vi "plcHMI_rev2.vi"() -> ()   [LabVIEW 2020]
doc: "ADS continuos synchronous write example using base blocks. \n\nThe client writes data synchronously and does wait for the respose from server."
uses:
  Agilent/AgilentTotalCluster.ctl
  Agilent/AgilentControl.ctl
  Agilent/Channel Config.ctl
  <vilib>/Platform/TimedLoop/XDataNode/timing_clust.ctl
  <vilib>/Platform/TimedLoop/XDataNode/nitl_modes.ctl
  <vilib>/Platform/TimedLoop/XDataNode/wakeup.ctl
  <userlib>/Beckhoff-LabVIEW-Interface/_DependsOn/With TypeResolving/Write Sync Single TypeResolved.vi
  <userlib>/Beckhoff-LabVIEW-Interface/_DependsOn/With TypeResolving/Read Sync Single TypeResolved.vi
  <vilib>/Platform/TimedLoop/XDataNode/XDataNode.xnode
  <vilib>/Platform/TimedLoop/XDataNode/XDNodeRunTimeDep.lvlib
panel:
  in  "Tab Control":T1(tab)
  out "error out":errorcluster
  in  "Symbol file path - MUST BE ENTERED\nLoad \"ADS Write AND Read Symbols REV X.X.xml\"":path
  out "bHasMached":bool
  out "Write Status":bool
  out "Read Status":bool
  in  "EXIT HMI":bool caption="STOP HMI\nEXIT HMI"
  out "Internal TwinCAT Handle ID Maps":dbl format="%#_12g"
  in  "802L TDK PSU Voltage Rating (abs(Volts))":i32=12000 min=1 max=50000
  in  "802L TDL PSU Peak Power (J/s)":i32=9000 min=1 max=50000
  in  "HVPS Model":u16(ring) items=["802L-12kV,9000J/s", "802L+50kV,9000J/s", "Other"]
  out "Test Interval Fault":bool
  in  "Cycle Time (Sec)":i32=15 min=0
  in  "Voltage Held by PSU":bool
  in  "Log Capacitor Voltage":bool
  in  "Log Temperature Data":bool
  out "Time Since Last Shot":string caption="Elapsed Time Text"
  in  "Duty Cycle":dbl
  in  "Current Control":bool
  out "Expected Voltage":i16
  in  "Dump":bool
  out "EOC":bool
  out "Maximum Test Number Reached":bool
  out "SCR Ready":bool
  in  "START":bool
  in  "STOP":bool
  in  "Hold":bool
  in  "Charge":bool
  in  "Shot":bool
  in  "HV Switch Mode":bool
  in  "CLEAR FAULT":bool
  in  "Manual/Auto":bool=TRUE
  out "Test Interval (Sec)":i32=15 min=0
  in  "Capacitance (uF)":sgl=1e-13 min=0 max=10000 format="%#_6f"
  in  "Target Charge Volt (V) - Min 1500V - TEMPORARY LIMIT 12kV":i32 min=-12000 max=12000 step=1
  out "Estimated Charge Time (seconds)":sgl
  in  "Hold Time Before Shot (seconds)":i16 min=0 max=1000
  in  "Max Number of Shots (Test intervals)":i32=1 min=1 max=999
  out "Shot Number":i32
  out "Charge Fault":bool=TRUE
  out "Discharge Fault":bool=TRUE
  out "Hold Fault":bool=TRUE
  out "Cap 1 Temp\nExceeded Fault":bool=TRUE
  out "Ambient Temp\nExceeded Fault":bool=TRUE
  out "PSU Fault":bool=TRUE
  out "Control Sys Fault":bool=TRUE
  out "test Running":bool
  out "Test State":string
  out "Cap 1 Voltage":i16
  out "Cap 1 Temperature":i16
  in  "Capacitor Voltage Data Log File Path (.xlsx)":path
  out "Load Temperature":i16
  out "Soft Dump Temp":i16
  out "Ambient Temp":i16
  out "Waveform Chart - Capacitor Voltage (Probe, abs(Volts))":dbl(graph)
  in  "Manual Charge Time (seconds)":sgl=-1.0 min=-1 max=90
  in  "Reset Test Number":bool
  in  "Cap 1 Fault Temp (Cel)":i16 min=0 max=125
  in  "Capacitor Temperature Data Log File Path (.xlsx)":path
  out "Cap 1 Voltage (HVPS)":i16
  out "Capacitor Voltage":cluster{dbl, dbl}(graph)
  out "EOC":i16(graph)
  out "Soft Exception":bool
  out "PSU HV FB Fault":bool
  out "Charge FB Fault":bool
  out "Softdump FB Fault":bool
  out "SCR FB":i16(graph)
  in  "CH4 Vertical Units":string(combo)="V"
  in  "CH4 Vertical Units/div":dbl=2.0
  in  "Toggle Scope Scale":bool
  in  "CH1 Vertical Units/div":dbl=2.0
  in  "CH1 Vertical Units":string(combo)="V"
  in  "Horizontal Units":enum16{"us", "ms", "s"}(ring)
  in  "Horizontal Units/div":dbl=200.0
  out "Download":bool
  in  "Single":bool
  in  "Stop":bool
  out "Scope Trig":bool
  in  "Agilent Array":T2[](array[typedef])
  out "Process Step":i32
  in  "C:\\HVTest\\Local_Cap_Log_Scope (.xlsx)":path
  out "Stop Loops":bool
  # "CONFIGURATION"
  # "Press STOP HMI instead of\nLabView Abort Execution"
  # "PSU V Rating, Peak Power\nactive when OTHER\nis selected"
  # "INPUT VARIABLES - For TDK Lambda 802L\nMust be written to before START"
  # "FAULT STATUSES"
  # "Set to -1 for automated\nfull charge to setpoint"
  # "MANUAL CONTROLS"
  # "Does not record during \"wait\" and appends to data file. Must be named with .xlsx"
  # "HV Switch Configuration"
  # "Records during \"Test Running.\" Must be named with .xlsx"
  # "Control Sys Faults"
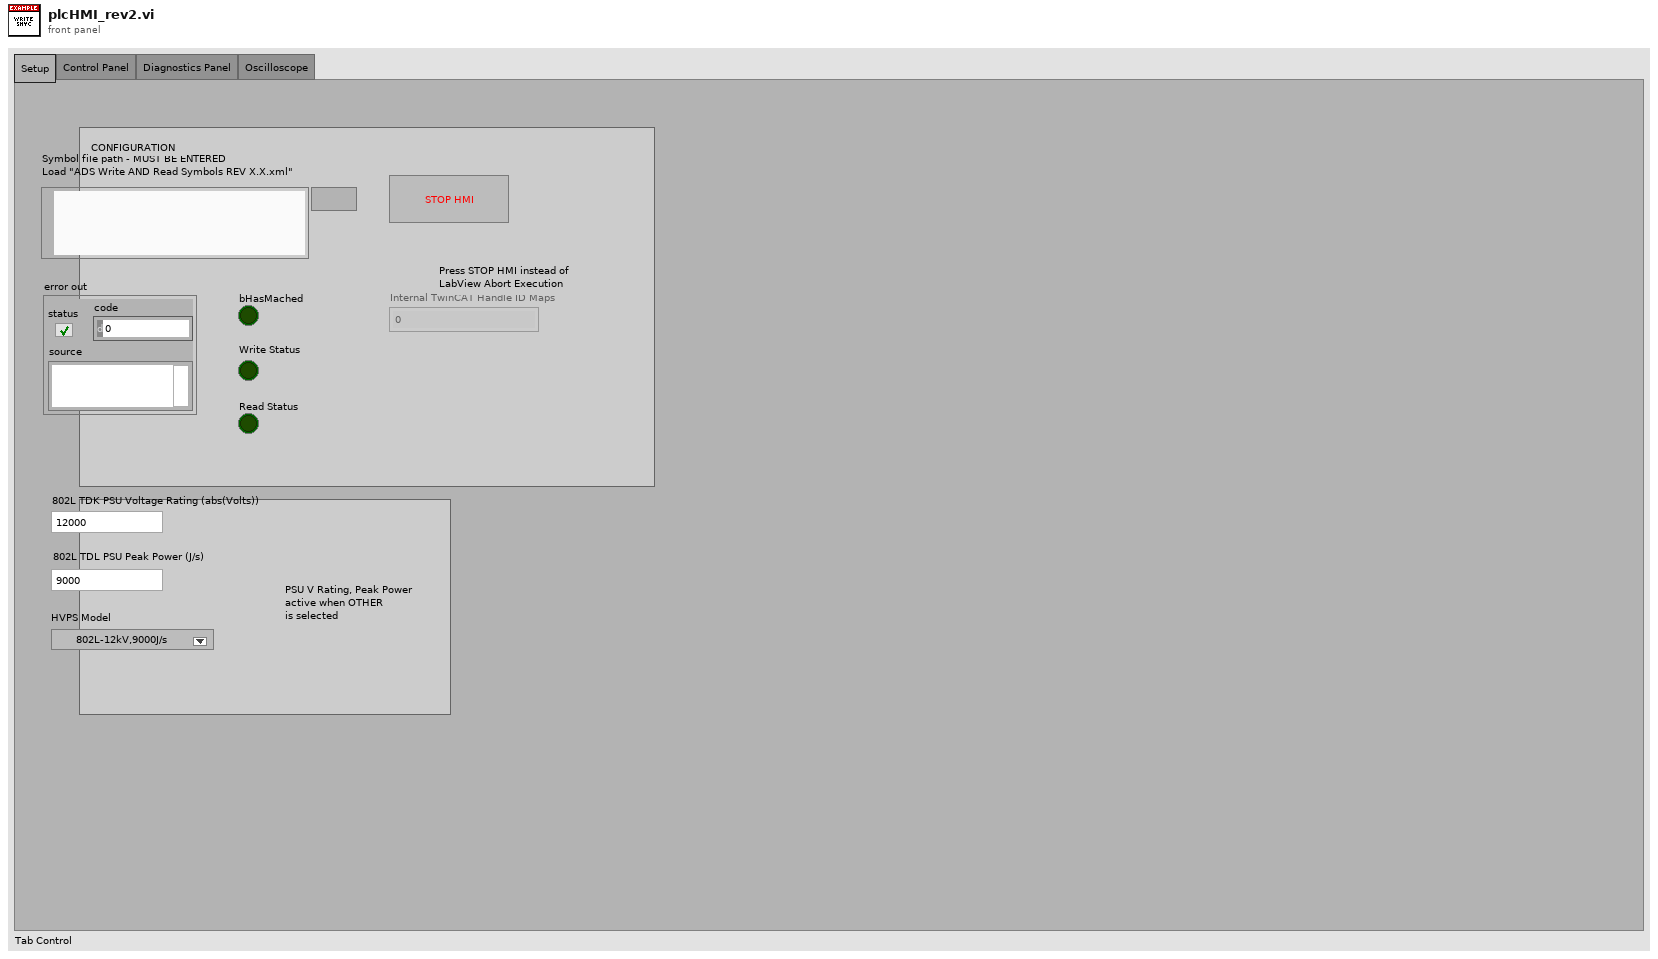
[diagram p1: front panel]
types:
  T1 = enum32{"Setup", "Control Panel", "Diagnostics Panel", "Oscilloscope"}
  T2 = typedef "AgilentTotalCluster.ctl" = cluster{"Agilent Graph":waveform(dbl)[], "Agilent Control":T3, "Agilent Setup Error":errorcluster, "Agilent Present":bool, "Enabled":bool}
  T3 = typedef "AgilentControl.ctl" = cluster{"Trig?":bool, "VISA session":refnum<visa-resource-name>, "Setup to Load":string, "Timeout (ms)":u32, "Desired Samp":enum32{"100", "250", "500", "1000", "2000", "5000", "10000", "20000", "50000", "100000", "200000", "500000", "1000000", "2000000", "4000000", "8000000"}, "Captured Samp":i32, "Desired Channels":T4[]}
  T4 = typedef "Channel Config.ctl" = cluster{"Chan Index":enum16{"Channel1", "Channel2", "Channel3", "Channel4", "MATH"}, "Name":string, "Samples":i32}
  T5 = typedef "XDNodeRunTimeDep.lvlib/timing_clust.ctl" = cluster{"Expected End [f-1]":u64, "Actual End [f-1]":u64, "Finished Late? [f-1]":bool, "Expected End [i-1]":u64, "Actual End [i-1]":u64, "Finished Late? [i-1]":bool, "Expected Start [i]":u64, "Actual Start [i]":u64, "Expected Start [f]":u64, "Actual Start [f]":u64, "Source Name":string, "Structure Name":string, "Period":i64, "Deadline":i64, "Offset":i64, "Start":i64, "Priority":i32, "Timeout":i32, "Mode":T6, "Wakeup Reason":T7, "Error":errorcluster, "Source Type":string, "Secondary Source Type":string, "Global End Time":u64, "Global Start Time":u64, "Frame Duration":u64, "Iteration Duration":u64, "Assigned CPU":i32, "I/O Scan Engine Mode":u32}
  T6 = typedef "XDNodeRunTimeDep.lvlib/nitl_modes.ctl" = enum32{"No Change", "Process missed periods, maintain original phase", "Discard missed periods, maintain original phase", "Process missed periods, ignore original phase", "Discard missed periods, ignore original phase"}
  T7 = typedef "XDNodeRunTimeDep.lvlib/wakeup.ctl" = enum32{"Normal", "Aborted", "Asynchronous wakeup", "Timing source error", "Timed loop error", "Timeout"}
  T8 = cluster{"Agilent Array[0]":T2, "Agilent Array[1]":T2, "Agilent Array[2]":T2, "Agilent Array[3]":T2, "Agilent Array[4]":T2, "Agilent Array[5]":T2, "Agilent Array[6]":T2, "Agilent Array[7]":T2, "Agilent Array[8]":T2}
  T9 = enum32{"100", "250", "500", "1000", "2000", "5000", "10000", "20000", "50000", "100000", "200000", "500000", "1000000", "2000000", "4000000", "8000000"}
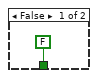
[diagram p2: hidden frame]
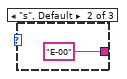
[diagram p5: hidden frame]
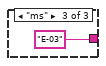
[diagram p6: hidden frame]
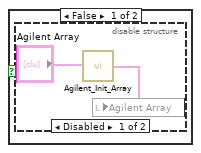
[diagram p7: hidden frame]
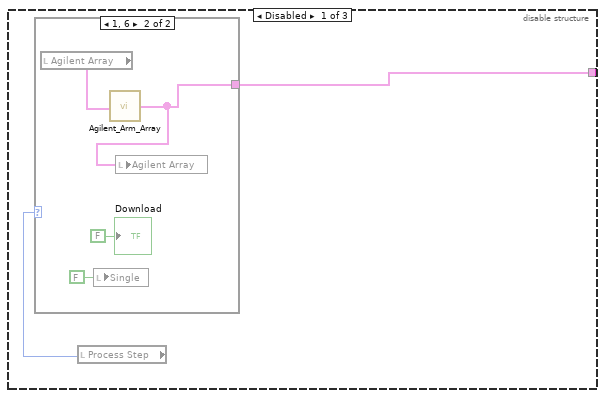
[diagram p11: hidden frame]
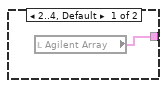
[diagram p12: hidden frame]
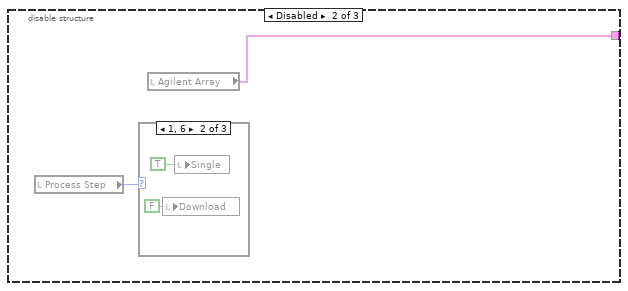
[diagram p13: hidden frame]
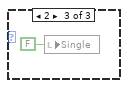
[diagram p15: hidden frame]
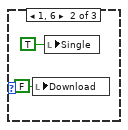
[diagram p17: hidden frame]
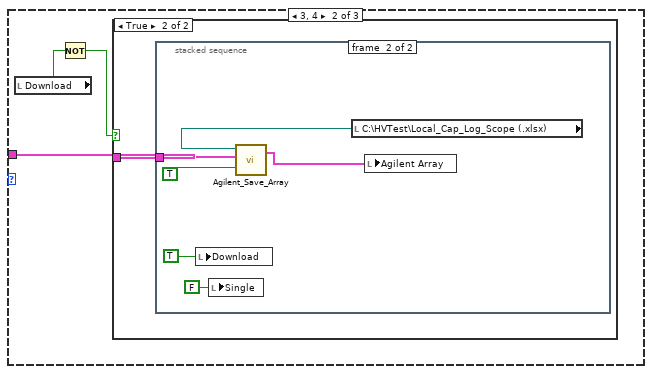
[diagram p19: hidden frame]
diagram:
  w95 = u16 17 items=["SyncLatest"=17, "AsyncLatest"=33] ("WriterMode")
  w188 = u16 33 items=["SyncLatest"=17, "AsyncLatest"=33] ("WriterMode")
  w227 = u16 33 items=["SyncLatest"=17, "AsyncLatest"=33] ("WriterMode")
  w246 = u16 33 items=["SyncLatest"=17, "AsyncLatest"=33] ("WriterMode")
  w265 = u16 33 items=["SyncLatest"=17, "AsyncLatest"=33] ("WriterMode")
  w284 = u16 33 items=["SyncLatest"=17, "AsyncLatest"=33] ("WriterMode")
  w303 = u16 33 items=["SyncLatest"=17, "AsyncLatest"=33] ("WriterMode")
  w322 = u16 33 items=["SyncLatest"=17, "AsyncLatest"=33] ("WriterMode")
  w341 = u16 17 items=["SyncLatest"=17, "AsyncLatest"=33] ("WriterMode")
  w360 = u16 17 items=["SyncLatest"=17, "AsyncLatest"=33] ("WriterMode")
  w379 = u16 17 items=["SyncLatest"=17, "AsyncLatest"=33] ("WriterMode")
  w398 = u16 17 items=["SyncLatest"=17, "AsyncLatest"=33] ("WriterMode")
  w417 = u16 17 items=["SyncLatest"=17, "AsyncLatest"=33] ("WriterMode")
  w436 = u16 17 items=["SyncLatest"=17, "AsyncLatest"=33] ("WriterMode")
  w455 = u16 17 items=["SyncLatest"=17, "AsyncLatest"=33] ("WriterMode")
  w470 = u16 17 items=["SyncLatest"=17, "AsyncLatest"=33] ("WriterMode")
  # "Variables/ Control"
  # "Documentation:\nCode separated vertically into two main sections - Write and read\nThey are further separated into BOOL and numeric\nThe OR gates wire all the error lines and the EXIT HMI button to a WHILE LOOP STOP\nThere current delay time on the routine is 100ms\nAll the AND gates connect the typecast resolve lines to the bHasMatched indicator\nThe second and third set of AND gates connect the write statuses to the Write Status indicator\nThe same is done for the read status indicator"
  # "WRITE NUMERICS"
  # "WRITE BOOLS"
  # "Select Symbol N"
  # "Read Initialization"
  # "Release \nTypeResolver"
  # "Release Writer"
  # "Send Request"
  # "Init \nTypeResolver"
  # "Init Writer"
  # "Select Symbol"
  # "Initialization"
  # "Call Release handle block\nat the end, when all nodes\nhave finished their execution"
  # "There must be only one release\nafter every init block.\nRelease block must be called\nalways at the end."
  # "Release"
  # "Symbol Interface"
  n1 = disable-structure shown="Enabled" {
    disable-tunnel: [w477 _] -> w475
    disable-tunnel: [w476 w479] -> w474
    frame Disabled {
      # "Using Symbol Interface"
      n2 = call <userlib>:"Symbol Interface.vi"() -> ("PortInfo"=w476:string, "error out"=w477:errorcluster)  [unwired: 14 in]
    }
    frame Enabled {
      # "Using Symbol File"
      n3 = Path To String(path="Symbol file path - MUST BE ENTERED\nLoad \"ADS Write AND Read Symbols REV X.X.xml\"") -> (string=w479:string)
    }
  }
  n4 = call <userlib>:"Init.vi"("XMLDescription"=w474, "error in (no error)"=w475) -> ("Handle"=w24:u32, "ReadGrpSymbols"=w5:string[], "WriteGrpSymbols"=w11:string[], "error out"=w16:errorcluster)  [unwired: 9 in, 1 out]
  n5 = Index Array(array=w11, index=21) -> (element=w10:string)
  n6 = Index Array(array=w11, index=20) -> (element=w17:string)
  n7 = Index Array(array=w11, index=14) -> (element=w228:string)
  n8 = Index Array(array=w11, index=9) -> (element=w323:string)
  n9 = Index Array(array=w11, index=10) -> (element=w304:string)
  n10 = Index Array(array=w11, index=12) -> (element=w266:string)
  n11 = Index Array(array=w11, index=11) -> (element=w285:string)
  n12 = Index Array(array=w11, index=13) -> (element=w247:string)
  n13 = Index Array(array=w11, index=18) -> (element=w25:string)
  n14 = Index Array(array=w11, index=19) -> (element=w18:string)
  n15 = Index Array(array=w11, index=7) -> (element=w342:string)
  n16 = Index Array(array=w11, index=2) -> (element=w437:string)
  n17 = Index Array(array=w11, index=3) -> (element=w418:string)
  n18 = Index Array(array=w11, index=5) -> (element=w380:string)
  n19 = Index Array(array=w11, index=4) -> (element=w399:string)
  n20 = Index Array(array=w11, index=6) -> (element=w361:string)
  n21 = Index Array(array=w11, index=1) -> (element=w456:string)
  n22 = Index Array(array=w11, index=16) -> (element=w122:string)
  n23 = Index Array(array=w11, index=8) -> (element=w94:string)
  n24 = Index Array(array=w11, index=0) -> (element=w471:string)
  n25 = Index Array(array=w11, index=15) -> (element=w189:string)
  n26 = Index Array(array=w11, index=17) -> (element=w78:string)
  n27 = call <userlib>:"Init Writer.vi"("Handle"=w24, "SymbolName"=w228, "WriterMode"=w227, "error constant"=w16) -> ("Handle"=w226:u32, "SymbolName"=w225:string, "WriterMode"=w224:u16, "WriteHandle"=w223:u32, "error IO"=w222:errorcluster)  [unwired: 7 in]
  n28 = call <userlib>:"Init Writer.vi"("Handle"=w24, "SymbolName"=w323, "WriterMode"=w322, "error constant"=w16) -> ("Handle"=w318:u32, "SymbolName"=w317:string, "WriterMode"=w316:u16, "WriteHandle"=w314:u32, "error IO"=w315:errorcluster)  [unwired: 7 in]
  n29 = call <userlib>:"Init Writer.vi"("Handle"=w24, "SymbolName"=w304, "WriterMode"=w303, "error constant"=w16) -> ("Handle"=w302:u32, "SymbolName"=w301:string, "WriterMode"=w300:u16, "WriteHandle"=w299:u32, "error IO"=w298:errorcluster)  [unwired: 7 in]
  n30 = call <userlib>:"Init Writer.vi"("Handle"=w24, "SymbolName"=w266, "WriterMode"=w265, "error constant"=w16) -> ("Handle"=w264:u32, "SymbolName"=w263:string, "WriterMode"=w262:u16, "WriteHandle"=w261:u32, "error IO"=w260:errorcluster)  [unwired: 7 in]
  n31 = call <userlib>:"Init Type.vi"("Handle"=w24, "SymbolName"=w228, "error in"=w16) -> ("Handle"=w221:u32, "TypeHdl"=w220:u32, "error IO"=w219:errorcluster)  [unwired: 7 in, 3 out]
  n32 = call <userlib>:"Init Type.vi"("Handle"=w24, "SymbolName"=w323, "error in"=w16) -> ("Handle"=w307:u32, "TypeHdl"=w306:u32, "error IO"=w305:errorcluster)  [unwired: 7 in, 3 out]
  n33 = call <userlib>:"Init Type.vi"("Handle"=w24, "SymbolName"=w304, "error in"=w16) -> ("Handle"=w297:u32, "TypeHdl"=w296:u32, "error IO"=w295:errorcluster)  [unwired: 7 in, 3 out]
  n34 = call <userlib>:"Init Writer.vi"("Handle"=w24, "SymbolName"=w285, "WriterMode"=w284, "error constant"=w16) -> ("Handle"=w283:u32, "SymbolName"=w282:string, "WriterMode"=w281:u16, "WriteHandle"=w280:u32, "error IO"=w279:errorcluster)  [unwired: 7 in]
  n35 = call <userlib>:"Init Type.vi"("Handle"=w24, "SymbolName"=w266, "error in"=w16) -> ("Handle"=w259:u32, "TypeHdl"=w258:u32, "error IO"=w257:errorcluster)  [unwired: 7 in, 3 out]
  n36 = call <userlib>:"Init Writer.vi"("Handle"=w24, "SymbolName"=w247, "WriterMode"=w246, "error constant"=w16) -> ("Handle"=w245:u32, "SymbolName"=w244:string, "WriterMode"=w243:u16, "WriteHandle"=w242:u32, "error IO"=w241:errorcluster)  [unwired: 7 in]
  n37 = call <userlib>:"Init Type.vi"("Handle"=w24, "SymbolName"=w285, "error in"=w16) -> ("Handle"=w278:u32, "TypeHdl"=w277:u32, "error IO"=w276:errorcluster)  [unwired: 7 in, 3 out]
  n38 = call <userlib>:"Init Type.vi"("Handle"=w24, "SymbolName"=w247, "error in"=w16) -> ("Handle"=w240:u32, "TypeHdl"=w239:u32, "error IO"=w238:errorcluster)  [unwired: 7 in, 3 out]
  n39 = call <userlib>:"Init Writer.vi"("Handle"=w24, "SymbolName"=w342, "WriterMode"=w341, "error constant"=w16) -> ("Handle"=w340:u32, "SymbolName"=w339:string, "WriterMode"=w338:u16, "WriteHandle"=w337:u32, "error IO"=w336:errorcluster)  [unwired: 7 in]
  n40 = call <userlib>:"Init Writer.vi"("Handle"=w24, "SymbolName"=w437, "WriterMode"=w436, "error constant"=w16) -> ("Handle"=w432:u32, "SymbolName"=w431:string, "WriterMode"=w430:u16, "WriteHandle"=w428:u32, "error IO"=w429:errorcluster)  [unwired: 7 in]
  n41 = call <userlib>:"Init Writer.vi"("Handle"=w24, "SymbolName"=w418, "WriterMode"=w417, "error constant"=w16) -> ("Handle"=w416:u32, "SymbolName"=w415:string, "WriterMode"=w414:u16, "WriteHandle"=w413:u32, "error IO"=w412:errorcluster)  [unwired: 7 in]
  n42 = call <userlib>:"Init Writer.vi"("Handle"=w24, "SymbolName"=w380, "WriterMode"=w379, "error constant"=w16) -> ("Handle"=w378:u32, "SymbolName"=w377:string, "WriterMode"=w376:u16, "WriteHandle"=w375:u32, "error IO"=w374:errorcluster)  [unwired: 7 in]
  n43 = call <userlib>:"Init Type.vi"("Handle"=w24, "SymbolName"=w342, "error in"=w16) -> ("Handle"=w335:u32, "TypeHdl"=w334:u32, "error IO"=w333:errorcluster)  [unwired: 7 in, 3 out]
  n44 = call <userlib>:"Init Type.vi"("Handle"=w24, "SymbolName"=w437, "error in"=w16) -> ("Handle"=w421:u32, "TypeHdl"=w420:u32, "error IO"=w419:errorcluster)  [unwired: 7 in, 3 out]
  n45 = call <userlib>:"Init Type.vi"("Handle"=w24, "SymbolName"=w418, "error in"=w16) -> ("Handle"=w411:u32, "TypeHdl"=w410:u32, "error IO"=w409:errorcluster)  [unwired: 7 in, 3 out]
  n46 = call <userlib>:"Init Writer.vi"("Handle"=w24, "SymbolName"=w399, "WriterMode"=w398, "error constant"=w16) -> ("Handle"=w397:u32, "SymbolName"=w396:string, "WriterMode"=w395:u16, "WriteHandle"=w394:u32, "error IO"=w393:errorcluster)  [unwired: 7 in]
  n47 = call <userlib>:"Init Type.vi"("Handle"=w24, "SymbolName"=w380, "error in"=w16) -> ("Handle"=w373:u32, "TypeHdl"=w372:u32, "error IO"=w371:errorcluster)  [unwired: 7 in, 3 out]
  n48 = call <userlib>:"Init Writer.vi"("Handle"=w24, "SymbolName"=w361, "WriterMode"=w360, "error constant"=w16) -> ("Handle"=w359:u32, "SymbolName"=w358:string, "WriterMode"=w357:u16, "WriteHandle"=w356:u32, "error IO"=w355:errorcluster)  [unwired: 7 in]
  n49 = call <userlib>:"Init Type.vi"("Handle"=w24, "SymbolName"=w399, "error in"=w16) -> ("Handle"=w392:u32, "TypeHdl"=w391:u32, "error IO"=w390:errorcluster)  [unwired: 7 in, 3 out]
  n50 = call <userlib>:"Init Type.vi"("Handle"=w24, "SymbolName"=w361, "error in"=w16) -> ("Handle"=w354:u32, "TypeHdl"=w353:u32, "error IO"=w352:errorcluster)  [unwired: 7 in, 3 out]
  n51 = call <userlib>:"Init Writer.vi"("Handle"=w24, "SymbolName"=w456, "WriterMode"=w455, "error constant"=w16) -> ("Handle"=w454:u32, "SymbolName"=w453:string, "WriterMode"=w452:u16, "WriteHandle"=w451:u32, "error IO"=w450:errorcluster)  [unwired: 7 in]
  n52 = call <userlib>:"Init Writer.vi"("Handle"=w24, "SymbolName"=w122, "error constant"=w16) -> ("Handle"=w121:u32, "SymbolName"=w120:string, "WriterMode"=w119:u16, "WriteHandle"=w117:u32, "error IO"=w118:errorcluster)  [unwired: 8 in]
  n53 = call <userlib>:"Init Type.vi"("Handle"=w24, "SymbolName"=w456, "error in"=w16) -> ("Handle"=w449:u32, "TypeHdl"=w448:u32, "error IO"=w447:errorcluster)  [unwired: 7 in, 3 out]
  n54 = call <userlib>:"Init Type.vi"("Handle"=w24, "SymbolName"=w122, "error in"=w16) -> ("Handle"=w116:u32, "TypeHdl"=w115:u32, "error IO"=w114:errorcluster)  [unwired: 7 in, 3 out]
  n55 = call <userlib>:"Init Writer.vi"("Handle"=w24, "SymbolName"=w471, "WriterMode"=w470, "error constant"=w16) -> ("Handle"=w469:u32, "SymbolName"=w468:string, "WriterMode"=w467:u16, "WriteHandle"=w466:u32, "error IO"=w465:errorcluster)  [unwired: 7 in]
  n56 = call <userlib>:"Init Type.vi"("Handle"=w24, "SymbolName"=w471, "error in"=w16) -> ("Handle"=w464:u32, "TypeHdl"=w463:u32, "error IO"=w458:errorcluster)  [unwired: 7 in, 3 out]
  n57 = call <userlib>:"Init Writer.vi"("Handle"=w24, "SymbolName"=w189, "WriterMode"=w188, "error constant"=w16) -> ("Handle"=w184:u32, "SymbolName"=w183:string, "WriterMode"=w182:u16, "WriteHandle"=w171:u32, "error IO"=w181:errorcluster)  [unwired: 7 in]
  n58 = call <userlib>:"Init Type.vi"("Handle"=w24, "SymbolName"=w189, "error in"=w16) -> ("Handle"=w177:u32, "TypeHdl"=w175:u32, "error IO"=w176:errorcluster)  [unwired: 7 in, 3 out]
  n59 = call <userlib>:"Init Writer.vi"("Handle"=w24, "SymbolName"=w78, "error constant"=w16) -> ("Handle"=w75:u32, "SymbolName"=w74:string, "WriterMode"=w73:u16, "WriteHandle"=w72:u32, "error IO"=w71:errorcluster)  [unwired: 8 in]
  n60 = call <userlib>:"Init Type.vi"("Handle"=w24, "SymbolName"=w78, "error in"=w16) -> ("Handle"=w70:u32, "TypeHdl"=w69:u32, "error IO"=w68:errorcluster)  [unwired: 7 in, 3 out]
  n61 = Index Array(array=w5, index=2) -> (element=w167:string)
  n62 = Index Array(array=w5, index=4) -> (element=w163:string)
  n63 = call <userlib>:"Init Writer.vi"("Handle"=w24, "SymbolName"=w94, "WriterMode"=w95, "error constant"=w16) -> ("Handle"=w93:u32, "SymbolName"=w92:string, "WriterMode"=w91:u16, "WriteHandle"=w90:u32, "error IO"=w89:errorcluster)  [unwired: 7 in]
  n64 = Index Array(array=w5, index=1) -> (element=w206:string)
  n65 = Index Array(array=w5, index=21) -> (element=w39:string)
  n66 = Index Array(array=w5, index=22) -> (element=w36:string)
  n67 = call <userlib>:"Init Type.vi"("Handle"=w24, "SymbolName"=w94, "error in"=w16) -> ("Handle"=w88:u32, "TypeHdl"=w87:u32, "error IO"=w86:errorcluster)  [unwired: 7 in, 3 out]
  n68 = Index Array(array=w5, index=0) -> (element=w205:string)
  n69 = Index Array(array=w5, index=3) -> (element=w164:string)
  n70 = Index Array(array=w5, index=20) -> (element=w44:string)
  n71 = Index Array(array=w5, index=23) -> (element=w35:string)
  n72 = Index Array(array=w5, index=16) -> (element=w169:string)
  n73 = Index Array(array=w5, index=24) -> (element=w33:string)
  n74 = Index Array(array=w5, index=11) -> (element=w194:string)
  n75 = Index Array(array=w5, index=10) -> (element=w195:string)
  n76 = Index Array(array=w5, index=17) -> (element=w47:string)
  n77 = Index Array(array=w5, index=18) -> (element=w46:string)
  n78 = Index Array(array=w5, index=13) -> (element=w192:string)
  n79 = Index Array(array=w5, index=27) -> (element=w3:string)
  n80 = Index Array(array=w5, index=12) -> (element=w193:string)
  n81 = Index Array(array=w5, index=15) -> (element=w190:string)
  n82 = Index Array(array=w5, index=19) -> (element=w45:string)
  n83 = Index Array(array=w5, index=26) -> (element=w4:string)
  n84 = Index Array(array=w5, index=5) -> (element=w59:string)
  n85 = Index Array(array=w5, index=6) -> (element=w157:string)
  n86 = Index Array(array=w5, index=9) -> (element=w204:string)
  n87 = Index Array(array=w5, index=14) -> (element=w191:string)
  n88 = Index Array(array=w5, index=8) -> (element=w159:string)
  n89 = Index Array(array=w5, index=25) -> (element=w22:string)
  n90 = Index Array(array=w5, index=7) -> (element=w158:string)
  n91 = node-c288(10) -> (w104:T5)  [unwired: 3 in]
  n92 = timed-loop {
    tunnel: w469 -> [w787]
    tunnel: w468 -> [w786]
    tunnel: w467 -> [w785]
    tunnel: w466 -> [w784]
    tunnel: w464 -> [w1061]
    tunnel: w463 -> [w1060]
    tunnel: [w782] -> w462
    tunnel: [w781] -> w461
    tunnel: [w1059] -> w460
    tunnel: [w1058] -> w459
    tunnel: w454 -> [w1056]
    tunnel: w453 -> [w1055]
    tunnel: w452 -> [w1054]
    tunnel: w451 -> [w1053]
    tunnel: w449 -> [w1051]
    tunnel: w448 -> [w1050]
    tunnel: [w1048] -> w445
    tunnel: [w1047] -> w444
    tunnel: [w1046] -> w442
    tunnel: [w1045] -> w441
    tunnel: w432 -> [w1044]
    tunnel: w431 -> [w1043]
    tunnel: w430 -> [w1042]
    tunnel: w428 -> [w1040]
    tunnel: [w1039] -> w427
    tunnel: [w1038] -> w426
    tunnel: [w1037] -> w423
    tunnel: [w1036] -> w422
    tunnel: w421 -> [w1035]
    tunnel: w420 -> [w1034]
    tunnel: w416 -> [w1032]
    tunnel: w415 -> [w1031]
    tunnel: w414 -> [w1030]
    tunnel: w413 -> [w1029]
    tunnel: w411 -> [w1027]
    tunnel: w410 -> [w1026]
    tunnel: [w1024] -> w407
    tunnel: [w1023] -> w406
    tunnel: [w1022] -> w404
    tunnel: [w1021] -> w403
    tunnel: w397 -> [w1020]
    tunnel: w396 -> [w1019]
    tunnel: w395 -> [w1018]
    tunnel: w394 -> [w1017]
    tunnel: w392 -> [w1015]
    tunnel: w391 -> [w1014]
    tunnel: [w1012] -> w388
    tunnel: [w1011] -> w387
    tunnel: [w1010] -> w385
    tunnel: [w1009] -> w384
    tunnel: w378 -> [w1008]
    tunnel: w377 -> [w1007]
    tunnel: w376 -> [w1006]
    tunnel: w375 -> [w1005]
    tunnel: w373 -> [w1003]
    tunnel: w372 -> [w1002]
    tunnel: [w1000] -> w369
    tunnel: [w999] -> w368
    tunnel: [w998] -> w366
    tunnel: [w997] -> w365
    tunnel: w359 -> [w996]
    tunnel: w358 -> [w995]
    tunnel: w357 -> [w994]
    tunnel: w356 -> [w993]
    tunnel: w354 -> [w991]
    tunnel: w353 -> [w990]
    tunnel: [w988] -> w350
    tunnel: [w987] -> w349
    tunnel: [w986] -> w347
    tunnel: [w985] -> w346
    tunnel: w340 -> [w984]
    tunnel: w339 -> [w983]
    tunnel: w338 -> [w982]
    tunnel: w337 -> [w981]
    tunnel: w335 -> [w979]
    tunnel: w334 -> [w978]
    tunnel: [w976] -> w331
    tunnel: [w975] -> w330
    tunnel: [w974] -> w328
    tunnel: [w973] -> w327
    tunnel: w318 -> [w972]
    tunnel: w317 -> [w971]
    tunnel: w316 -> [w970]
    tunnel: w314 -> [w968]
    tunnel: [w967] -> w313
    tunnel: [w966] -> w312
    tunnel: [w965] -> w309
    tunnel: [w964] -> w308
    tunnel: w307 -> [w963]
    tunnel: w306 -> [w962]
    tunnel: w302 -> [w960]
    tunnel: w301 -> [w959]
    tunnel: w300 -> [w958]
    tunnel: w299 -> [w957]
    tunnel: w297 -> [w955]
    tunnel: w296 -> [w954]
    tunnel: [w952] -> w293
    tunnel: [w951] -> w292
    tunnel: [w950] -> w290
    tunnel: [w949] -> w289
    tunnel: w283 -> [w948]
    tunnel: w282 -> [w947]
    tunnel: w281 -> [w946]
    tunnel: w280 -> [w945]
    tunnel: w278 -> [w943]
    tunnel: w277 -> [w942]
    tunnel: [w940] -> w274
    tunnel: [w939] -> w273
    tunnel: [w938] -> w271
    tunnel: [w937] -> w270
    tunnel: w264 -> [w936]
    tunnel: w263 -> [w935]
    tunnel: w262 -> [w934]
    tunnel: w261 -> [w933]
    tunnel: w259 -> [w931]
    tunnel: w258 -> [w930]
    tunnel: [w928] -> w255
    tunnel: [w927] -> w254
    tunnel: [w926] -> w252
    tunnel: [w925] -> w251
    tunnel: w245 -> [w924]
    tunnel: w244 -> [w923]
    tunnel: w243 -> [w922]
    tunnel: w242 -> [w921]
    tunnel: w240 -> [w919]
    tunnel: w239 -> [w918]
    tunnel: [w916] -> w236
    tunnel: [w915] -> w235
    tunnel: [w914] -> w233
    tunnel: [w913] -> w232
    tunnel: w226 -> [w912]
    tunnel: w225 -> [w911]
    tunnel: w224 -> [w910]
    tunnel: w223 -> [w909]
    tunnel: w221 -> [w907]
    tunnel: w220 -> [w906]
    tunnel: [w904] -> w217
    tunnel: [w903] -> w216
    tunnel: [w902] -> w214
    tunnel: [w901] -> w213
    tunnel: w206 -> [w900]
    tunnel: w205 -> [w899]
    tunnel: w204 -> [w898]
    tunnel: [w897] -> w152
    tunnel: w195 -> [w896]
    tunnel: w194 -> [w895]
    tunnel: w193 -> [w894]
    tunnel: w192 -> [w893]
    tunnel: w191 -> [w892]
    tunnel: w190 -> [w891]
    tunnel: [w890] -> w100
    tunnel: [w889] -> w151
    tunnel: [w888] -> w150
    tunnel: [w887] -> w149
    tunnel: [w886] -> w148
    tunnel: [w828] -> w147
    tunnel: [w826] -> w146
    shift-right: [w710] -> w473
    shift-left: w465 -> [w783]
    shift-right: [w709] -> w472
    shift-left: w458 -> [w1057]
    shift-right: [w707] -> w443
    shift-left: w450 -> [w1052]
    shift-right: [w706] -> w440
    shift-left: w447 -> [w1049]
    shift-right: [w704] -> w425
    shift-left: w429 -> [w1041]
    shift-right: [w703] -> w424
    shift-left: w419 -> [w1033]
    shift-right: [w701] -> w405
    shift-left: w412 -> [w1028]
    shift-right: [w700] -> w402
    shift-left: w409 -> [w1025]
    shift-right: [w698] -> w386
    shift-left: w393 -> [w1016]
    shift-right: [w697] -> w383
    shift-left: w390 -> [w1013]
    shift-right: [w695] -> w367
    shift-left: w374 -> [w1004]
    shift-right: [w694] -> w364
    shift-left: w371 -> [w1001]
    shift-right: [w692] -> w348
    shift-left: w355 -> [w992]
    shift-right: [w691] -> w345
    shift-left: w352 -> [w989]
    shift-right: [w689] -> w329
    shift-left: w336 -> [w980]
    shift-right: [w688] -> w326
    shift-left: w333 -> [w977]
    shift-right: [w687] -> w311
    shift-left: w315 -> [w969]
    shift-right: [w686] -> w310
    shift-left: w305 -> [w961]
    shift-right: [w684] -> w291
    shift-left: w298 -> [w956]
    shift-right: [w683] -> w288
    shift-left: w295 -> [w953]
    shift-right: [w681] -> w272
    shift-left: w279 -> [w944]
    shift-right: [w680] -> w269
    shift-left: w276 -> [w941]
    shift-right: [w678] -> w253
    shift-left: w260 -> [w932]
    shift-right: [w677] -> w250
    shift-left: w257 -> [w929]
    shift-right: [w675] -> w234
    shift-left: w241 -> [w920]
    shift-right: [w674] -> w231
    shift-left: w238 -> [w917]
    shift-right: [w672] -> w215
    shift-left: w222 -> [w908]
    shift-right: [w671] -> w212
    shift-left: w219 -> [w905]
    tunnel: w184 -> [w868]
    tunnel: w183 -> [w867]
    tunnel: w182 -> [w866]
    tunnel: w181 -> [w865]
    tunnel: [w669] -> w180
    tunnel: [w864] -> w179
    tunnel: [w863] -> w178
    tunnel: w177 -> [w862]
    tunnel: w176 -> [w861]
    tunnel: w175 -> [w860]
    tunnel: [w668] -> w174
    tunnel: [w859] -> w173
    tunnel: [w858] -> w172
    tunnel: w171 -> [w857]
    tunnel: w169 -> [w856]
    tunnel: [w827] -> w145
    tunnel: [w850] -> w154
    tunnel: w16 -> [w849]
    tunnel: [w847] -> w153
    tunnel: w167 -> [w846]
    tunnel: w164 -> [w842]
    tunnel: w163 -> [w841]
    tunnel: [w832] -> w155
    tunnel: [w831] -> w156
    tunnel: w159 -> [w825]
    tunnel: w158 -> [w824]
    tunnel: w157 -> [w823]
    tunnel: [w810] -> w56
    tunnel: [w809] -> w55
    tunnel: [w808] -> w54
    tunnel: w121 -> [w801]
    tunnel: w120 -> [w800]
    tunnel: w119 -> [w799]
    tunnel: w118 -> [w798]
    tunnel: w117 -> [w797]
    tunnel: w116 -> [w795]
    tunnel: w115 -> [w794]
    tunnel: w114 -> [w793]
    tunnel: [w792] -> w111
    tunnel: [w791] -> w110
    tunnel: [w666] -> w109
    tunnel: [w665] -> w108
    tunnel: [w790] -> w107
    tunnel: [w789] -> w106
    timing: w104 -> [_]
    timing-out: [_] -> w103
    tunnel: w24 -> [w780]
    tunnel: [w663] -> w58
    tunnel: w93 -> [w658]
    tunnel: w92 -> [w657]
    tunnel: w91 -> [w656]
    tunnel: w90 -> [w655]
    tunnel: w89 -> [w654]
    tunnel: w88 -> [w653]
    tunnel: w87 -> [w652]
    tunnel: w86 -> [w651]
    tunnel: [w649] -> w85
    tunnel: [w648] -> w84
    tunnel: [w641] -> w83
    tunnel: [w640] -> w82
    tunnel: [w647] -> w81
    tunnel: [w646] -> w80
    tunnel: w75 -> [w634]
    tunnel: w74 -> [w633]
    tunnel: w73 -> [w632]
    tunnel: w72 -> [w631]
    tunnel: w71 -> [w630]
    tunnel: w70 -> [w629]
    tunnel: w69 -> [w628]
    tunnel: w68 -> [w627]
    tunnel: [w625] -> w67
    tunnel: [w622] -> w66
    tunnel: [w617] -> w65
    tunnel: [w616] -> w64
    tunnel: [w624] -> w63
    tunnel: [w623] -> w62
    tunnel: [w615] -> w57
    tunnel: w59 -> [w611]
    tunnel: [w610] -> w53
    tunnel: w47 -> [w605]
    tunnel: w46 -> [w600]
    tunnel: w45 -> [w599]
    tunnel: w44 -> [w598]
    tunnel: [w595] -> w43
    tunnel: [w593] -> w42
    tunnel: [w588] -> w41
    tunnel: [w587] -> w28
    tunnel: w39 -> [w585]
    tunnel: w36 -> [w560]
    tunnel: w35 -> [w559]
    tunnel: w33 -> [w552]
    tunnel: [w548] -> w32
    tunnel: [w547] -> w31
    tunnel: [w546] -> w30
    tunnel: [w545] -> w29
    tunnel: w25 -> [w544]
    tunnel: w24 -> [w506]
    tunnel: w16 -> [w543]
    tunnel: [w538] -> w15
    tunnel: [w537] -> _
    tunnel: w22 -> [w533]
    tunnel: [w529] -> w21
    tunnel: w18 -> [w528]
    tunnel: w17 -> [w527]
    tunnel: w16 -> [w502]
    tunnel: [w522] -> w14
    tunnel: [w521] -> w13
    tunnel: w10 -> [w507]
    tunnel: [w501] -> w9
    tunnel: w4 -> [w488]
    tunnel: w3 -> [w487]
    tunnel: [w482] -> w2
    tunnel: [w481] -> w1
    stop <- w606 stop-if-true
    # "Stop Loop on Error (OR gates)"
    # "Error Stop Loop AND"
    # "Typecast Match AND"
    # "Write Status AND"
    # "READ BOOLS"
    # "READ NUMERICS"
    # "STOP HMI via error or EXIT button"
    # "Check Read status and\nthen convert Variant \nto LabVIEW type (AND gates)"
    # "Sync Read Single"
    n93 = node-c288() -> (w664:errorcluster)  [unwired: 1 in]
    n94 = disable-structure shown="Enabled" {
      frame Enabled {
        n95 = flat-sequence {
          tunnel: [w1201] -> w1145
          tunnel: w1145 -> [w1220]
          frame #0 {
            n96 = disable-structure shown="Enabled" {
              frame Enabled {
                n97 = feedback #1(TRUE) -> (w1147:bool)
                n98 = And(x=TRUE, y=w1147) -> (x .and. y?=w1150:bool)
                n99 = case shown="True" w1150 {
                  tunnel: [FALSE FALSE] -> w1148
                  frame False {
                  }
                  frame True {
                    n100 = local read "Agilent Array"() -> (w1153:T2[])
                    n101 = call "Agilent_Init_Array.vi"("Agilent Array In"=w1153) -> ("Agilent Array Out"=w1154:T2[])
                    n102 = call "Agilent_Arm_Array.vi"("Agilent Array In"=w1154) -> ("Agilent Array Out"=w1152:T2[])
                    n103 = local write "Agilent Array"(w1152) -> ()
                  }
                }
                n104 = feedback-in #1(w1148) -> ()
              }
              frame Disabled {
              }
            }
          }
          frame #1 {
            n105 = case shown="True" "Toggle Scope Scale" {
              frame False {
              }
              frame True {
                n106 = Number To Decimal String(number="CH4 Vertical Units/div") -> (decimal integer string=w1160:string)  [unwired: 1 in]
                n107 = Number To Decimal String(number="Horizontal Units/div") -> (decimal integer string=w1168:string)  [unwired: 1 in]
                n108 = Number To Decimal String(number="CH1 Vertical Units/div") -> (decimal integer string=w1166:string)  [unwired: 1 in]
                n109 = case shown="\"us\"" "Horizontal Units" {
                  tunnel: ["E-06" "E-00" "E-03"] -> w1177
                  frame "us" {
                  }
                  frame "s", Default {
                  }
                  frame "ms" {
                  }
                }
                n110 = Concatenate Strings(":CHAN4:SCAL " ("write buffer"), w1160, "CH4 Vertical Units") -> (w1159:string)
                n111 = Concatenate Strings(":CHAN1:SCAL " ("write buffer"), w1166, "CH1 Vertical Units") -> (w1173:string)
                n112 = Concatenate Strings(":TIM:SCAL " ("write buffer"), w1168, w1177) -> (w1176:string)
                n113 = VISA Open(VISA resource name=refnum<visa-resource-name> "HV_Test_Scope") -> (VISA resource name=w1171:refnum<visa-resource-name>, error out=w1172:errorcluster)  [unwired: 4 in]
                n114 = VISA Write(VISA resource name=w1171, write buffer=w1176, error in (no error)=w1172) -> (VISA resource name out=w1180:refnum<visa-resource-name>, error out=w1179:errorcluster)  [unwired: 1 out]
                n115 = VISA Write(VISA resource name=w1180, write buffer=w1173, error in (no error)=w1179) -> (VISA resource name out=w1165:refnum<visa-resource-name>, error out=w1163:errorcluster)  [unwired: 1 out]
                n116 = VISA Write(VISA resource name=w1165, write buffer=w1159, error in (no error)=w1163) -> (VISA resource name out=w1164:refnum<visa-resource-name>, error out=w1162:errorcluster)  [unwired: 1 out]
                n117 = VISA Close(VISA resource name=w1164, error in (no error)=w1162) -> ()  [unwired: 1 out]
              }
            }
          }
          frame #2 {
            n118 = disable-structure shown="Enabled" {
              frame Enabled {
                n119 = case shown="True" "Stop" {
                  frame False {
                    n120 = disable-structure shown="Disabled" {
                      frame Disabled {
                        n121 = call "Agilent_Init_Array.vi"("Agilent Array In"="Agilent Array") -> ("Agilent Array Out"=w1187:T2[])
                        n122 = local write "Agilent Array"(w1187) -> ()
                      }
                      frame Enabled {
                      }
                    }
                  }
                  frame True {
                    n123 = VISA Open(VISA resource name=refnum<visa-resource-name> "HV_Test_Scope") -> (VISA resource name=w1193:refnum<visa-resource-name>, error out=w1194:errorcluster)  [unwired: 4 in]
                    n124 = VISA Write(VISA resource name=w1193, write buffer=":STOP", error in (no error)=w1194) -> (VISA resource name out=w1191:refnum<visa-resource-name>, error out=w1192:errorcluster)  [unwired: 1 out]
                    n125 = VISA Close(VISA resource name=w1191, error in (no error)=w1192) -> ()  [unwired: 1 out]
                  }
                }
              }
              frame Disabled {
              }
            }
            n126 = case shown="True" "Single" {
              frame False {
              }
              frame True {
                n127 = VISA Open(VISA resource name=refnum<visa-resource-name> "HV_Test_Scope") -> (VISA resource name=w1199:refnum<visa-resource-name>, error out=w1200:errorcluster)  [unwired: 4 in]
                n128 = VISA Write(VISA resource name=w1199, write buffer=":SINGLE", error in (no error)=w1200) -> (VISA resource name out=w1197:refnum<visa-resource-name>, error out=w1198:errorcluster)  [unwired: 1 out]
                n129 = VISA Close(VISA resource name=w1197, error in (no error)=w1198) -> ()  [unwired: 1 out]
              }
            }
          }
          frame #3 {
            n130 = disable-structure shown="Enabled" {
              disable-tunnel: [w1203 w1210 w1215] -> w1201
              frame Disabled {
                n131 = local read "Process Step"() -> (w1202:i32)
                n132 = case shown="1, 6" w1202 {
                  tunnel: [w1204 w1208] -> w1203
                  frame 2..4, Default {
                    n133 = local read "Agilent Array"() -> (w1204:T2[])
                  }
                  frame 1, 6 {
                    n134 = local read "Agilent Array"() -> (w1205:T2[])
                    n135 = local write "Single"(FALSE ("Single")) -> ()
                    n136 = call "Agilent_Arm_Array.vi"("Agilent Array In"=w1205) -> ("Agilent Array Out"=w1208:T2[])
                    n137 = local write "Agilent Array"(w1208) -> ()
                    "Download" <- FALSE ("Downloading")
                  }
                }
              }
              frame Disabled {
                n138 = local read "Process Step"() -> (w1209:i32)
                n139 = case shown="1, 6" w1209 {
                  frame 0, Default {
                  }
                  frame 1, 6 {
                    n140 = local write "Download"(FALSE ("Download")) -> ()
                    n141 = local write "Single"(TRUE ("Single")) -> ()
                  }
                  frame 2 {
                    n142 = local write "Single"(FALSE ("Single")) -> ()
                  }
                }
                n143 = local read "Agilent Array"() -> (w1210:T2[])
              }
              frame Enabled {
                n144 = local read "Process Step"() -> (w1214:i32)
                n145 = case shown="2, 7" w1214 {
                  frame 0, Default {
                  }
                  frame 1, 6 {
                    n146 = local write "Download"(FALSE ("Download")) -> ()
                    n147 = local write "Single"(TRUE ("Single")) -> ()
                  }
                  frame 2, 7 {
                    n148 = local write "Single"(FALSE ("Single")) -> ()
                  }
                }
                n149 = local read "Agilent Array"() -> (w1215:T2[])
              }
            }
          }
          frame #4 {
            n150 = local read "Process Step"() -> (w1219:i32)
            n151 = case shown="0" w1219 {
              tunnel: w1220 -> [_ w1223 w1236]
              frame Default {
              }
              frame 3, 4 {
                n152 = local read "Download"() -> (w1222:bool)
                n153 = Not(x=w1222) -> (.not. x?=w1221:bool)
                n154 = case shown="True" w1221 {
                  tunnel: w1223 -> [_ w1224]
                  frame False {
                  }
                  frame True {
                    n155 = stacked-sequence {
                      tunnel: w1224 -> [_ w1234]
                      frame #0 {
                        n156 = local read "Agilent Array"() -> (w1228:T2[])
                        n157 = Array To Cluster(array=w1228) -> (cluster=w1227:T8)
                        n158 = Unbundle By Name(w1227) -> ("Agilent Array[0].Agilent Control.Desired Samp"=w1225:T9)
                        n159 = call "GF_SetRecordLengthProperly.vi"("Num Samples"=w1225, "VISA resource name"=refnum<visa-resource-name> "HV_Test_Scope") -> ()  [unwired: 1 in, 2 out]
                      }
                      frame #1 {
                        n160 = local write "Download"(TRUE ("Downloading")) -> ()
                        n161 = local write "Single"(FALSE ("Single")) -> ()
                        n162 = local read "C:\\HVTest\\Local_Cap_Log_Scope (.xlsx)"() -> (w1229:path)
                        n163 = call "Agilent_Save_Array.vi"("Agilent Download"=TRUE, "Agilent Array In"=w1234, "File Path"=w1229) -> ("Agilent Array Out"=w1232:T2[])  [unwired: 1 in, 1 out]
                        n164 = local write "Agilent Array"(w1232) -> ()
                      }
                    }
                  }
                }
              }
              frame 0 {
                n165 = local read "Maximum Test Number Reached"() -> (w1235:bool)
                n166 = case shown="True" w1235 {
                  tunnel: w1236 -> [_ w1239]
                  frame False {
                  }
                  frame True {
                    n167 = local read "Download"() -> (w1238:bool)
                    n168 = Not(x=w1238) -> (.not. x?=w1237:bool)
                    n169 = case shown="True" w1237 {
                      tunnel: w1239 -> [_ w1240]
                      frame False {
                      }
                      frame True {
                        n170 = stacked-sequence {
                          tunnel: w1240 -> [_ w1250]
                          frame #0 {
                            n171 = local read "Agilent Array"() -> (w1244:T2[])
                            n172 = Array To Cluster(array=w1244) -> (cluster=w1243:T8)
                            n173 = Unbundle By Name(w1243) -> ("Agilent Array[0].Agilent Control.Desired Samp"=w1241:T9)
                            n174 = call "GF_SetRecordLengthProperly.vi"("Num Samples"=w1241, "VISA resource name"=refnum<visa-resource-name> "HV_Test_Scope") -> ()  [unwired: 1 in, 2 out]
                          }
                          frame #1 {
                            n175 = local write "Download"(TRUE ("Downloading")) -> ()
                            n176 = local write "Single"(FALSE ("Single")) -> ()
                            n177 = call "Agilent_Save_Array.vi"("Agilent Download"=TRUE, "Agilent Array In"=w1250, "File Path"="C:\\HVTest\\Local_Cap_Log_Scope (.xlsx)") -> ("Agilent Array Out"=w1248:T2[])  [unwired: 1 in, 1 out]
                            n178 = local write "Agilent Array"(w1248) -> ()
                          }
                        }
                      }
                    }
                  }
                }
              }
            }
          }
        }
      }
      frame Disabled {
      }
    }
    n179 = case shown="0, Default" "HVPS Model" {
      tunnel: ["802L TDK PSU Voltage Rating (abs(Volts))" 12000 50000] -> w788
      tunnel: ["802L TDL PSU Peak Power (J/s)" 9000 9000] -> w829
      frame 2 {
      }
      frame 0, Default {
      }
      frame 1 {
      }
    }
    n180 = flat-sequence {
      tunnel: w629 -> [w1271]
      tunnel: w628 -> [w1272]
      tunnel: w627 -> [w1269]
      tunnel: [w1269] -> w638
      tunnel: [w1272] -> w637
      tunnel: [w1271] -> w636
      tunnel: [w1270] -> w635
      tunnel: [w1275] -> w616
      tunnel: [w1278] -> w623
      tunnel: [w1277] -> w624
      tunnel: [w1276] -> w626
      tunnel: w638 -> [w1281]
      tunnel: w637 -> [w1280]
      tunnel: w636 -> [w1279]
      tunnel: w635 -> [w1274]
      tunnel: [w1273] -> w540
      frame #0 {
        # "Write Data"
        n181 = To Word Integer(number="Cap 1 Fault Temp (Cel)") -> (16bit integer=w1267:i16)
        n182 = To Variant(anything=w1267) -> (Variant=w1270:variant)
      }
      frame #1 {
        # "Resolve To TC"
        n183 = call <userlib>:"Resolve To TC Type.vi"("Handle"=w1279, "TypHdl"=w1280, "WData"=w1274, "error in"=w1281) -> ("Handle"=w1277:u32, "TypHdl"=w1278:u32, "bHasMatched"=w1273:bool, "ADSWData"=w1276:variant, "error out"=w1275:errorcluster)  [unwired: 7 in]
      }
    }
    n184 = flat-sequence {
      tunnel: w907 -> [w1483]
      tunnel: w906 -> [w1484]
      tunnel: w905 -> [w1485]
      tunnel: [w1485] -> w1089
      tunnel: [w1484] -> w1088
      tunnel: [w1483] -> w1087
      tunnel: [w1482] -> w1086
      tunnel: [w1488] -> w671
      tunnel: [w1491] -> w901
      tunnel: [w1490] -> w902
      tunnel: [w1489] -> w874
      tunnel: w1089 -> [w1494]
      tunnel: w1088 -> [w1493]
      tunnel: w1087 -> [w1492]
      tunnel: w1086 -> [w1487]
      tunnel: [w1486] -> w735
      frame #0 {
        # "Write Data"
        n185 = To Long Integer(number="Max Number of Shots (Test intervals)") -> (32bit integer=w1481:i32)
        n186 = To Variant(anything=w1481) -> (Variant=w1482:variant)
      }
      frame #1 {
        # "Resolve To TC"
        n187 = call <userlib>:"Resolve To TC Type.vi"("Handle"=w1492, "TypHdl"=w1493, "WData"=w1487, "error in"=w1494) -> ("Handle"=w1490:u32, "TypHdl"=w1491:u32, "bHasMatched"=w1486:bool, "ADSWData"=w1489:variant, "error out"=w1488:errorcluster)  [unwired: 7 in]
      }
    }
    n188 = flat-sequence {
      tunnel: w862 -> [w1378]
      tunnel: w860 -> [w1379]
      tunnel: w861 -> [w1380]
      tunnel: [w1380] -> w873
      tunnel: [w1379] -> w872
      tunnel: [w1378] -> w871
      tunnel: [w1377] -> w870
      tunnel: w829 -> [w1375]
      tunnel: [w1383] -> w668
      tunnel: [w1386] -> w858
      tunnel: [w1385] -> w859
      tunnel: [w1384] -> w869
      tunnel: w873 -> [w1389]
      tunnel: w872 -> [w1388]
      tunnel: w871 -> [w1387]
      tunnel: w870 -> [w1382]
      tunnel: [w1381] -> w737
      frame #0 {
        # "Write Data"
        n189 = To Long Integer(number=w1375) -> (32bit integer=w1376:i32)
        n190 = To Variant(anything=w1376) -> (Variant=w1377:variant)
      }
      frame #1 {
        # "Resolve To TC"
        n191 = call <userlib>:"Resolve To TC Type.vi"("Handle"=w1387, "TypHdl"=w1388, "WData"=w1382, "error in"=w1389) -> ("Handle"=w1385:u32, "TypHdl"=w1386:u32, "bHasMatched"=w1381:bool, "ADSWData"=w1384:variant, "error out"=w1383:errorcluster)  [unwired: 7 in]
      }
    }
    n192 = flat-sequence {
      tunnel: w795 -> [w1358]
      tunnel: w794 -> [w1359]
      tunnel: w793 -> [w1356]
      tunnel: [w1356] -> w805
      tunnel: [w1359] -> w804
      tunnel: [w1358] -> w803
      tunnel: [w1357] -> w802
      tunnel: [w1362] -> w665
      tunnel: [w1365] -> w790
      tunnel: [w1364] -> w789
      tunnel: [w1363] -> w796
      tunnel: w805 -> [w1368]
      tunnel: w804 -> [w1367]
      tunnel: w803 -> [w1366]
      tunnel: w802 -> [w1361]
      tunnel: [w1360] -> w621
      frame #0 {
        # "Write Data"
        n193 = To Single Precision Float(number="Manual Charge Time (seconds)") -> (single precision float=w1354:sgl)
        n194 = To Variant(anything=w1354) -> (Variant=w1357:variant)
      }
      frame #1 {
        # "Resolve To TC"
        n195 = call <userlib>:"Resolve To TC Type.vi"("Handle"=w1366, "TypHdl"=w1367, "WData"=w1361, "error in"=w1368) -> ("Handle"=w1364:u32, "TypHdl"=w1365:u32, "bHasMatched"=w1360:bool, "ADSWData"=w1363:variant, "error out"=w1362:errorcluster)  [unwired: 7 in]
      }
    }
    n196 = flat-sequence {
      tunnel: w955 -> [w1543]
      tunnel: w954 -> [w1544]
      tunnel: w953 -> [w1545]
      tunnel: [w1545] -> w1105
      tunnel: [w1544] -> w1104
      tunnel: [w1543] -> w1103
      tunnel: [w1542] -> w1102
      tunnel: [w1548] -> w683
      tunnel: [w1551] -> w949
      tunnel: [w1550] -> w950
      tunnel: [w1549] -> w878
      tunnel: w1105 -> [w1554]
      tunnel: w1104 -> [w1553]
      tunnel: w1103 -> [w1552]
      tunnel: w1102 -> [w1547]
      tunnel: [w1546] -> w727
      frame #0 {
        # "Write Data"
        n197 = To Single Precision Float(number="Capacitance (uF)") -> (single precision float=w1541:sgl)
        n198 = To Variant(anything=w1541) -> (Variant=w1542:variant)
      }
      frame #1 {
        # "Resolve To TC"
        n199 = call <userlib>:"Resolve To TC Type.vi"("Handle"=w1552, "TypHdl"=w1553, "WData"=w1547, "error in"=w1554) -> ("Handle"=w1550:u32, "TypHdl"=w1551:u32, "bHasMatched"=w1546:bool, "ADSWData"=w1549:variant, "error out"=w1548:errorcluster)  [unwired: 7 in]
      }
    }
    n200 = flat-sequence {
      tunnel: w931 -> [w1513]
      tunnel: w930 -> [w1514]
      tunnel: w929 -> [w1515]
      tunnel: [w1515] -> w1097
      tunnel: [w1514] -> w1096
      tunnel: [w1513] -> w1095
      tunnel: [w1512] -> w1094
      tunnel: w788 -> [w1510]
      tunnel: [w1518] -> w677
      tunnel: [w1521] -> w925
      tunnel: [w1520] -> w926
      tunnel: [w1519] -> w876
      tunnel: w1097 -> [w1524]
      tunnel: w1096 -> [w1523]
      tunnel: w1095 -> [w1522]
      tunnel: w1094 -> [w1517]
      tunnel: [w1516] -> w731
      frame #0 {
        # "Write Data"
        n201 = To Long Integer(number=w1510) -> (32bit integer=w1511:i32)
        n202 = To Variant(anything=w1511) -> (Variant=w1512:variant)
      }
      frame #1 {
        # "Resolve To TC"
        n203 = call <userlib>:"Resolve To TC Type.vi"("Handle"=w1522, "TypHdl"=w1523, "WData"=w1517, "error in"=w1524) -> ("Handle"=w1520:u32, "TypHdl"=w1521:u32, "bHasMatched"=w1516:bool, "ADSWData"=w1519:variant, "error out"=w1518:errorcluster)  [unwired: 7 in]
      }
    }
    n204 = flat-sequence {
      tunnel: w963 -> [w1559]
      tunnel: [w1557] -> _
      tunnel: w961 -> [w1560]
      tunnel: [w1560] -> w1109
      tunnel: [w1557] -> w1108
      tunnel: [w1559] -> w1107
      tunnel: [w1558] -> w1106
      tunnel: w962 -> [w1557]
      tunnel: [w1563] -> w686
      tunnel: [w1566] -> w965
      tunnel: [w1565] -> w964
      tunnel: [w1564] -> w879
      tunnel: w1109 -> [w1569]
      tunnel: w1108 -> [w1568]
      tunnel: w1107 -> [w1567]
      tunnel: w1106 -> [w1562]
      tunnel: [w1561] -> w725
      frame #0 {
        # "Write Data"
        n205 = To Long Integer(number="Cycle Time (Sec)") -> (32bit integer=w1556:i32)
        n206 = To Variant(anything=w1556) -> (Variant=w1558:variant)
      }
      frame #1 {
        # "Resolve To TC"
        n207 = call <userlib>:"Resolve To TC Type.vi"("Handle"=w1567, "TypHdl"=w1568, "WData"=w1562, "error in"=w1569) -> ("Handle"=w1565:u32, "TypHdl"=w1566:u32, "bHasMatched"=w1561:bool, "ADSWData"=w1564:variant, "error out"=w1563:errorcluster)  [unwired: 7 in]
      }
    }
    n208 = flat-sequence {
      tunnel: w943 -> [w1528]
      tunnel: w942 -> [w1529]
      tunnel: w941 -> [w1530]
      tunnel: [w1530] -> w1101
      tunnel: [w1529] -> w1100
      tunnel: [w1528] -> w1099
      tunnel: [w1527] -> w1098
      tunnel: [w1533] -> w680
      tunnel: [w1536] -> w937
      tunnel: [w1535] -> w938
      tunnel: [w1534] -> w877
      tunnel: w1101 -> [w1539]
      tunnel: w1100 -> [w1538]
      tunnel: w1099 -> [w1537]
      tunnel: w1098 -> [w1532]
      tunnel: [w1531] -> w729
      frame #0 {
        # "Write Data"
        n209 = To Long Integer(number="Target Charge Volt (V) - Min 1500V - TEMPORARY LIMIT 12kV") -> (32bit integer=w1526:i32)
        n210 = To Variant(anything=w1526) -> (Variant=w1527:variant)
      }
      frame #1 {
        # "Resolve To TC"
        n211 = call <userlib>:"Resolve To TC Type.vi"("Handle"=w1537, "TypHdl"=w1538, "WData"=w1532, "error in"=w1539) -> ("Handle"=w1535:u32, "TypHdl"=w1536:u32, "bHasMatched"=w1531:bool, "ADSWData"=w1534:variant, "error out"=w1533:errorcluster)  [unwired: 7 in]
      }
    }
    n212 = flat-sequence {
      tunnel: w919 -> [w1498]
      tunnel: w918 -> [w1499]
      tunnel: w917 -> [w1500]
      tunnel: [w1500] -> w1093
      tunnel: [w1499] -> w1092
      tunnel: [w1498] -> w1091
      tunnel: [w1497] -> w1090
      tunnel: [w1503] -> w674
      tunnel: [w1506] -> w913
      tunnel: [w1505] -> w914
      tunnel: [w1504] -> w875
      tunnel: w1093 -> [w1509]
      tunnel: w1092 -> [w1508]
      tunnel: w1091 -> [w1507]
      tunnel: w1090 -> [w1502]
      tunnel: [w1501] -> w733
      frame #0 {
        # "Write Data"
        n213 = To Word Integer(number="Hold Time Before Shot (seconds)") -> (16bit integer=w1496:i16)
        n214 = To Variant(anything=w1496) -> (Variant=w1497:variant)
      }
      frame #1 {
        # "Resolve To TC"
        n215 = call <userlib>:"Resolve To TC Type.vi"("Handle"=w1507, "TypHdl"=w1508, "WData"=w1502, "error in"=w1509) -> ("Handle"=w1505:u32, "TypHdl"=w1506:u32, "bHasMatched"=w1501:bool, "ADSWData"=w1504:variant, "error out"=w1503:errorcluster)  [unwired: 7 in]
      }
    }
    n216 = flat-sequence {
      tunnel: w979 -> [w1393]
      tunnel: w978 -> [w1394]
      tunnel: w977 -> [w1395]
      tunnel: [w1395] -> w1065
      tunnel: [w1394] -> w1064
      tunnel: [w1393] -> w1063
      tunnel: [w1392] -> w1062
      tunnel: [w1398] -> w688
      tunnel: [w1401] -> w973
      tunnel: [w1400] -> w974
      tunnel: [w1399] -> w880
      tunnel: w1065 -> [w1404]
      tunnel: w1064 -> [w1403]
      tunnel: w1063 -> [w1402]
      tunnel: w1062 -> [w1397]
      tunnel: [w1396] -> w724
      frame #0 {
        # "Write Data"
        n217 = And(x="CLEAR FAULT", y="CLEAR FAULT") -> (x .and. y?=w1391:bool)
        n218 = To Variant(anything=w1391) -> (Variant=w1392:variant)
      }
      frame #1 {
        # "Resolve To TC"
        n219 = call <userlib>:"Resolve To TC Type.vi"("Handle"=w1402, "TypHdl"=w1403, "WData"=w1397, "error in"=w1404) -> ("Handle"=w1400:u32, "TypHdl"=w1401:u32, "bHasMatched"=w1396:bool, "ADSWData"=w1399:variant, "error out"=w1398:errorcluster)  [unwired: 7 in]
      }
    }
    n220 = flat-sequence {
      tunnel: w1027 -> [w1453]
      tunnel: w1026 -> [w1454]
      tunnel: w1025 -> [w1455]
      tunnel: [w1455] -> w1081
      tunnel: [w1454] -> w1080
      tunnel: [w1453] -> w1079
      tunnel: [w1452] -> w1078
      tunnel: [w1458] -> w700
      tunnel: [w1461] -> w1021
      tunnel: [w1460] -> w1022
      tunnel: [w1459] -> w884
      tunnel: w1081 -> [w1464]
      tunnel: w1080 -> [w1463]
      tunnel: w1079 -> [w1462]
      tunnel: w1078 -> [w1457]
      tunnel: [w1456] -> w716
      frame #0 {
        # "Write Data"
        n221 = And(x="Hold", y="Hold") -> (x .and. y?=w1451:bool)
        n222 = To Variant(anything=w1451) -> (Variant=w1452:variant)
      }
      frame #1 {
        # "Resolve To TC"
        n223 = call <userlib>:"Resolve To TC Type.vi"("Handle"=w1462, "TypHdl"=w1463, "WData"=w1457, "error in"=w1464) -> ("Handle"=w1460:u32, "TypHdl"=w1461:u32, "bHasMatched"=w1456:bool, "ADSWData"=w1459:variant, "error out"=w1458:errorcluster)  [unwired: 7 in]
      }
    }
    n224 = flat-sequence {
      tunnel: w1003 -> [w1423]
      tunnel: w1002 -> [w1424]
      tunnel: w1001 -> [w1425]
      tunnel: [w1425] -> w1073
      tunnel: [w1424] -> w1072
      tunnel: [w1423] -> w1071
      tunnel: [w1422] -> w1070
      tunnel: [w1428] -> w694
      tunnel: [w1431] -> w997
      tunnel: [w1430] -> w998
      tunnel: [w1429] -> w882
      tunnel: w1073 -> [w1434]
      tunnel: w1072 -> [w1433]
      tunnel: w1071 -> [w1432]
      tunnel: w1070 -> [w1427]
      tunnel: [w1426] -> w720
      frame #0 {
        # "Write Data"
        n225 = And(x="Shot", y="Shot") -> (x .and. y?=w1421:bool)
        n226 = To Variant(anything=w1421) -> (Variant=w1422:variant)
      }
      frame #1 {
        # "Resolve To TC"
        n227 = call <userlib>:"Resolve To TC Type.vi"("Handle"=w1432, "TypHdl"=w1433, "WData"=w1427, "error in"=w1434) -> ("Handle"=w1430:u32, "TypHdl"=w1431:u32, "bHasMatched"=w1426:bool, "ADSWData"=w1429:variant, "error out"=w1428:errorcluster)  [unwired: 7 in]
      }
    }
    n228 = flat-sequence {
      tunnel: w1035 -> [w1469]
      tunnel: [w1465] -> _
      tunnel: w1033 -> [w1470]
      tunnel: [w1470] -> w1085
      tunnel: [w1465] -> w1084
      tunnel: [w1469] -> w1083
      tunnel: [w1468] -> w1082
      tunnel: w1034 -> [w1465]
      tunnel: [w1473] -> w703
      tunnel: [w1476] -> w1037
      tunnel: [w1475] -> w1036
      tunnel: [w1474] -> w885
      tunnel: w1085 -> [w1479]
      tunnel: w1084 -> [w1478]
      tunnel: w1083 -> [w1477]
      tunnel: w1082 -> [w1472]
      tunnel: [w1471] -> w714
      frame #0 {
        # "Write Data"
        n229 = And(x="Manual/Auto", y="Manual/Auto") -> (x .and. y?=w1467:bool)
        n230 = To Variant(anything=w1467) -> (Variant=w1468:variant)
      }
      frame #1 {
        # "Resolve To TC"
        n231 = call <userlib>:"Resolve To TC Type.vi"("Handle"=w1477, "TypHdl"=w1478, "WData"=w1472, "error in"=w1479) -> ("Handle"=w1475:u32, "TypHdl"=w1476:u32, "bHasMatched"=w1471:bool, "ADSWData"=w1474:variant, "error out"=w1473:errorcluster)  [unwired: 7 in]
      }
    }
    n232 = flat-sequence {
      tunnel: w1015 -> [w1438]
      tunnel: w1014 -> [w1439]
      tunnel: w1013 -> [w1440]
      tunnel: [w1440] -> w1077
      tunnel: [w1439] -> w1076
      tunnel: [w1438] -> w1075
      tunnel: [w1437] -> w1074
      tunnel: [w1443] -> w697
      tunnel: [w1446] -> w1009
      tunnel: [w1445] -> w1010
      tunnel: [w1444] -> w883
      tunnel: w1077 -> [w1449]
      tunnel: w1076 -> [w1448]
      tunnel: w1075 -> [w1447]
      tunnel: w1074 -> [w1442]
      tunnel: [w1441] -> w718
      frame #0 {
        # "Write Data"
        n233 = And(x="Charge", y="Charge") -> (x .and. y?=w1436:bool)
        n234 = To Variant(anything=w1436) -> (Variant=w1437:variant)
      }
      frame #1 {
        # "Resolve To TC"
        n235 = call <userlib>:"Resolve To TC Type.vi"("Handle"=w1447, "TypHdl"=w1448, "WData"=w1442, "error in"=w1449) -> ("Handle"=w1445:u32, "TypHdl"=w1446:u32, "bHasMatched"=w1441:bool, "ADSWData"=w1444:variant, "error out"=w1443:errorcluster)  [unwired: 7 in]
      }
    }
    n236 = flat-sequence {
      tunnel: w991 -> [w1408]
      tunnel: w990 -> [w1409]
      tunnel: w989 -> [w1410]
      tunnel: [w1410] -> w1069
      tunnel: [w1409] -> w1068
      tunnel: [w1408] -> w1067
      tunnel: [w1407] -> w1066
      tunnel: [w1413] -> w691
      tunnel: [w1416] -> w985
      tunnel: [w1415] -> w986
      tunnel: [w1414] -> w881
      tunnel: w1069 -> [w1419]
      tunnel: w1068 -> [w1418]
      tunnel: w1067 -> [w1417]
      tunnel: w1066 -> [w1412]
      tunnel: [w1411] -> w722
      frame #0 {
        # "Write Data"
        n237 = And(x="HV Switch Mode", y="HV Switch Mode") -> (x .and. y?=w1406:bool)
        n238 = To Variant(anything=w1406) -> (Variant=w1407:variant)
      }
      frame #1 {
        # "Resolve To TC"
        n239 = call <userlib>:"Resolve To TC Type.vi"("Handle"=w1417, "TypHdl"=w1418, "WData"=w1412, "error in"=w1419) -> ("Handle"=w1415:u32, "TypHdl"=w1416:u32, "bHasMatched"=w1411:bool, "ADSWData"=w1414:variant, "error out"=w1413:errorcluster)  [unwired: 7 in]
      }
    }
    n240 = flat-sequence {
      tunnel: w1051 -> [w1339]
      tunnel: w1050 -> [w1340]
      tunnel: w1049 -> [w1341]
      tunnel: [w1341] -> w779
      tunnel: [w1340] -> w778
      tunnel: [w1339] -> w777
      tunnel: [w1338] -> w776
      tunnel: w779 -> [w1350]
      tunnel: w778 -> [w1349]
      tunnel: w777 -> [w1348]
      tunnel: w776 -> [w1343]
      tunnel: [w1344] -> w706
      tunnel: [w1347] -> w1045
      tunnel: [w1346] -> w1046
      tunnel: [w1345] -> w775
      tunnel: [w1342] -> w712
      frame #0 {
        # "Write Data"
        n241 = And(x="STOP", y="STOP") -> (x .and. y?=w1337:bool)
        n242 = To Variant(anything=w1337) -> (Variant=w1338:variant)
      }
      frame #1 {
        # "Resolve To TC"
        n243 = call <userlib>:"Resolve To TC Type.vi"("Handle"=w1348, "TypHdl"=w1349, "WData"=w1343, "error in"=w1350) -> ("Handle"=w1346:u32, "TypHdl"=w1347:u32, "bHasMatched"=w1342:bool, "ADSWData"=w1345:variant, "error out"=w1344:errorcluster)  [unwired: 7 in]
      }
    }
    n244 = flat-sequence {
      tunnel: w653 -> [w1286]
      tunnel: w652 -> [w1282]
      tunnel: w651 -> [w1287]
      tunnel: [w1287] -> w662
      tunnel: [w1282] -> w661
      tunnel: [w1286] -> w660
      tunnel: [w1285] -> w659
      tunnel: [w1290] -> w640
      tunnel: [w1293] -> w646
      tunnel: [w1292] -> w647
      tunnel: [w1291] -> w650
      tunnel: w662 -> [w1296]
      tunnel: w661 -> [w1295]
      tunnel: w660 -> [w1294]
      tunnel: w659 -> [w1289]
      tunnel: [w1288] -> w644
      frame #0 {
        # "Write Data"
        n245 = And(x="Reset Test Number", y="Reset Test Number") -> (x .and. y?=w1284:bool)
        n246 = To Variant(anything=w1284) -> (Variant=w1285:variant)
      }
      frame #1 {
        # "Resolve To TC"
        n247 = call <userlib>:"Resolve To TC Type.vi"("Handle"=w1294, "TypHdl"=w1295, "WData"=w1289, "error in"=w1296) -> ("Handle"=w1292:u32, "TypHdl"=w1293:u32, "bHasMatched"=w1288:bool, "ADSWData"=w1291:variant, "error out"=w1290:errorcluster)  [unwired: 7 in]
      }
    }
    n248 = flat-sequence {
      tunnel: w1061 -> [w1305]
      tunnel: w1060 -> [w1306]
      tunnel: w1057 -> [w1307]
      tunnel: [w1307] -> w774
      tunnel: [w1306] -> w773
      tunnel: [w1305] -> w772
      tunnel: [w1304] -> w771
      tunnel: [w1302] -> _
      tunnel: [w1302] -> w770
      tunnel: w787 -> [w1302]
      tunnel: w786 -> [w1301]
      tunnel: [w1301] -> w769
      tunnel: w785 -> [w1300]
      tunnel: [w1300] -> w768
      tunnel: w784 -> [w1299]
      tunnel: [w1299] -> w767
      tunnel: w783 -> [w1298]
      tunnel: [w1298] -> w766
      tunnel: ["START"] -> w562
      tunnel: w774 -> [w1321]
      tunnel: w773 -> [w1320]
      tunnel: w772 -> [w1319]
      tunnel: w771 -> [w1314]
      tunnel: [w1315] -> w765
      tunnel: [w1318] -> w764
      tunnel: [w1317] -> w763
      tunnel: [w1316] -> w762
      tunnel: [w1313] -> w761
      tunnel: w770 -> [w1312]
      tunnel: [w1312] -> w760
      tunnel: w769 -> [w1311]
      tunnel: [w1311] -> w759
      tunnel: w768 -> [w1310]
      tunnel: [w1310] -> w758
      tunnel: w767 -> [w1309]
      tunnel: [w1309] -> w757
      tunnel: [w1308] -> w756
      tunnel: w766 -> [w1308]
      tunnel: [w1332] -> w739
      tunnel: [w1333] -> w1059
      tunnel: [w1334] -> w1058
      tunnel: [w1335] -> w709
      tunnel: w765 -> [w1335]
      tunnel: w764 -> [w1334]
      tunnel: w763 -> [w1333]
      tunnel: w762 -> [w1324]
      tunnel: w761 -> [w1332]
      tunnel: w760 -> [w1331]
      tunnel: w759 -> [w1330]
      tunnel: w758 -> [w1329]
      tunnel: w757 -> [w1328]
      tunnel: w756 -> [w1327]
      tunnel: [w1326] -> w782
      tunnel: [w1325] -> w781
      tunnel: [w1323] -> w710
      tunnel: [w1322] -> w754
      frame #0 {
        # "Write Data"
        n249 = And(x="START", y="START") -> (x .and. y?=w1303:bool)
        n250 = To Variant(anything=w1303) -> (Variant=w1304:variant)
      }
      frame #1 {
        # "Resolve To TC"
        n251 = call <userlib>:"Resolve To TC Type.vi"("Handle"=w1319, "TypHdl"=w1320, "WData"=w1314, "error in"=w1321) -> ("Handle"=w1317:u32, "TypHdl"=w1318:u32, "bHasMatched"=w1313:bool, "ADSWData"=w1316:variant, "error out"=w1315:errorcluster)  [unwired: 7 in]
      }
      frame #2 {
        # "Write"
        n252 = call <userlib>:"Send Writer-Request.vi"("Handle"=w1331, "SymbolName"=w1330, "WriterMode"=w1329, "WriteHandle"=w1328, "error constant"=w1327, "ADS Write Data"=w1324) -> ("Handle"=w1326:u32, "WriteHandle"=w1325:u32, "Write status?"=w1322:bool, "error IO"=w1323:errorcluster)  [unwired: 5 in, 1 out]
      }
    }
    n253 = To Single Precision Float(number="Duty Cycle") -> (single precision float=w519:sgl)
    n254 = And(x="Voltage Held by PSU", y="Voltage Held by PSU") -> (x .and. y?=w505:bool)
    n255 = And(x="Current Control", y="Current Control") -> (x .and. y?=w526:bool)
    n256 = To Variant(anything=w519) -> (Variant=w523:variant)
    n257 = And(x="Dump", y="Dump") -> (x .and. y?=w535:bool)
    n258 = To Variant(anything=w505) -> (Variant=w503:variant)
    n259 = To Variant(anything=w526) -> (Variant=w524:variant)
    n260 = To Variant(anything=w535) -> (Variant=w536:variant)
    n261 = call-poly <userlib>:"Write TypeResolved.vi"("Handle"=w506, "SymbolName"=w507, "WData"=w503, "error constant"=w502) -> ("Write Status?"=w495:bool, "Has Matched?"=w496:bool, "error out"=w501:errorcluster)  [unwired: 8 in, 1 out]
    n262 = call-poly <userlib>:"Write TypeResolved.vi"("Handle"=w506, "SymbolName"=w527, "WData"=w523, "error constant"=w502) -> ("Write Status?"=w494:bool, "Has Matched?"=w497:bool, "error out"=w521:errorcluster)  [unwired: 8 in, 1 out]
    n263 = call-poly <userlib>:"Write TypeResolved.vi"("Handle"=w506, "SymbolName"=w528, "WData"=w524, "error constant"=w502) -> ("Write Status?"=w493:bool, "Has Matched?"=w498:bool, "error out"=w522:errorcluster)  [unwired: 8 in, 1 out]
    n264 = call <userlib>:"Send Writer-Request.vi"("Handle"=w1056, "SymbolName"=w1055, "WriterMode"=w1054, "WriteHandle"=w1053, "error constant"=w1052, "ADS Write Data"=w775) -> ("Handle"=w1048:u32, "WriteHandle"=w1047:u32, "Write status?"=w753:bool, "error IO"=w707:errorcluster)  [unwired: 5 in, 1 out]
    n265 = flat-sequence {
      tunnel: w900 -> [w1700]
      tunnel: w899 -> [w1698]
      tunnel: w898 -> [w1696]
      tunnel: [w1699] -> w1144
      tunnel: [w1697] -> w1143
      tunnel: [w1695] -> w1142
      tunnel: [w1694] -> w1141
      tunnel: [w1693] -> w1140
      tunnel: [w1692] -> w1139
      tunnel: [w1691] -> w1138
      tunnel: [w1690] -> w1137
      tunnel: [w1689] -> w1136
      tunnel: [w1688] -> w1135
      tunnel: [w1687] -> w1134
      tunnel: w896 -> [w1686]
      tunnel: w895 -> [w1685]
      tunnel: w894 -> [w1684]
      tunnel: w893 -> [w1683]
      tunnel: w892 -> [w1682]
      tunnel: w891 -> [w1681]
      tunnel: [w1680] -> w1133
      tunnel: [w1679] -> w1132
      tunnel: [w1678] -> w1131
      tunnel: [w1677] -> w1130
      tunnel: [w1676] -> w1129
      tunnel: [w1675] -> w1128
      tunnel: [w1674] -> w1127
      tunnel: [w1673] -> w1126
      tunnel: [w1672] -> w1125
      tunnel: [w1671] -> w1124
      tunnel: [w1670] -> w1123
      tunnel: [w1669] -> w1122
      tunnel: [w1668] -> w1121
      tunnel: [w1667] -> w1120
      tunnel: [w1666] -> w1119
      tunnel: [w1665] -> w1118
      tunnel: [w1664] -> w1117
      tunnel: [w1663] -> w1116
      tunnel: [w1662] -> w1115
      tunnel: [w1661] -> w1114
      tunnel: [w1660] -> w1113
      tunnel: [w1659] -> w1112
      tunnel: [w1658] -> w1111
      tunnel: [w1657] -> w1110
      tunnel: w856 -> [w1656]
      tunnel: [w1655] -> w855
      tunnel: [w1654] -> w854
      tunnel: [w1653] -> w853
      tunnel: [w1652] -> w852
      tunnel: [w1651] -> w851
      tunnel: w849 -> [w1582]
      tunnel: [w1650] -> w848
      tunnel: w846 -> [w1649]
      tunnel: [w1648] -> w845
      tunnel: [w1647] -> w844
      tunnel: [w1646] -> w843
      tunnel: w842 -> [w1645]
      tunnel: w841 -> [w1644]
      tunnel: [w1643] -> w840
      tunnel: [w1642] -> w839
      tunnel: [w1641] -> w838
      tunnel: [w1640] -> w837
      tunnel: [w1639] -> w836
      tunnel: [w1638] -> w835
      tunnel: [w1637] -> w834
      tunnel: [w1636] -> w833
      tunnel: w825 -> [w1635]
      tunnel: w824 -> [w1634]
      tunnel: w823 -> [w1633]
      tunnel: [w1632] -> w822
      tunnel: [w1631] -> w821
      tunnel: [w1630] -> w820
      tunnel: [w1629] -> w819
      tunnel: [w1628] -> w818
      tunnel: [w1627] -> w817
      tunnel: [w1626] -> w816
      tunnel: [w1625] -> w815
      tunnel: [w1624] -> w814
      tunnel: [w1623] -> w813
      tunnel: [w1622] -> w812
      tunnel: [w1621] -> w811
      tunnel: [w1573] -> _
      tunnel: w780 -> [w1573]
      tunnel: [w1620] -> w614
      tunnel: [w1619] -> w613
      tunnel: [w1618] -> w612
      tunnel: w611 -> [w1617]
      tunnel: [w1616] -> w607
      tunnel: w605 -> [w1615]
      tunnel: [w1614] -> w604
      tunnel: [w1613] -> w603
      tunnel: [w1612] -> w602
      tunnel: [w1611] -> w601
      tunnel: w600 -> [w1610]
      tunnel: w599 -> [w1609]
      tunnel: w598 -> [w1608]
      tunnel: [w1607] -> w597
      tunnel: [w1606] -> w596
      tunnel: [w1605] -> w594
      tunnel: [w1604] -> w592
      tunnel: [w1603] -> w591
      tunnel: [w1602] -> w590
      tunnel: [w1601] -> w589
      tunnel: [w1600] -> w586
      tunnel: w585 -> [w1599]
      tunnel: [w1598] -> w584
      tunnel: [w1597] -> w583
      tunnel: [w1596] -> w582
      tunnel: w560 -> [w1595]
      tunnel: w559 -> [w1594]
      tunnel: [w1593] -> w558
      tunnel: [w1592] -> w557
      tunnel: [w1591] -> w556
      tunnel: [w1590] -> w555
      tunnel: [w1589] -> w554
      tunnel: [w1588] -> w553
      tunnel: w552 -> [w1587]
      tunnel: [w1586] -> w551
      tunnel: [w1585] -> w550
      tunnel: [w1584] -> w549
      tunnel: w533 -> [w1583]
      tunnel: [w1581] -> w532
      tunnel: [w1580] -> w531
      tunnel: [w1579] -> w530
      tunnel: [w1578] -> w490
      tunnel: [w1577] -> w489
      tunnel: w488 -> [w1576]
      tunnel: w487 -> [w1574]
      tunnel: [w1575] -> w486
      tunnel: [w1572] -> w485
      tunnel: [w1571] -> w484
      tunnel: [w1570] -> w483
      tunnel: w1144 -> [w1889]
      tunnel: w1143 -> [w1902]
      tunnel: w1142 -> [_]
      tunnel: w1141 -> [w1888]
      tunnel: w1140 -> [w1887]
      tunnel: w1139 -> [w1903]
      tunnel: [w1804] -> w897
      tunnel: w1138 -> [w1901]
      tunnel: w1137 -> [w1904]
      tunnel: w1136 -> [w1906]
      tunnel: w1135 -> [w1864]
      tunnel: w1134 -> [_]
      tunnel: w1133 -> [w1884]
      tunnel: w1132 -> [w1899]
      tunnel: w1131 -> [w1897]
      tunnel: w1130 -> [w1895]
      tunnel: w1129 -> [w1893]
      tunnel: w1128 -> [w1891]
      tunnel: [w1817] -> w890
      tunnel: w1127 -> [w1883]
      tunnel: w1126 -> [w1882]
      tunnel: w1125 -> [w1881]
      tunnel: w1124 -> [w1880]
      tunnel: w1123 -> [w1879]
      tunnel: w1122 -> [w1878]
      tunnel: w1121 -> [_]
      tunnel: w1120 -> [w1877]
      tunnel: w1119 -> [_]
      tunnel: w1118 -> [w1876]
      tunnel: w1117 -> [_]
      tunnel: w1116 -> [w1875]
      tunnel: w1115 -> [_]
      tunnel: w1114 -> [w1874]
      tunnel: w1113 -> [_]
      tunnel: w1112 -> [w1873]
      tunnel: w1111 -> [_]
      tunnel: w1110 -> [w1872]
      tunnel: [w1819] -> w889
      tunnel: [w1821] -> w888
      tunnel: [w1823] -> w887
      tunnel: [w1825] -> w886
      tunnel: w855 -> [w1862]
      tunnel: w854 -> [w1861]
      tunnel: w853 -> [_]
      tunnel: w852 -> [w1787]
      tunnel: w851 -> [w1856]
      tunnel: [w1808] -> w850
      tunnel: w848 -> [w1860]
      tunnel: [w1806] -> w847
      tunnel: w845 -> [w1859]
      tunnel: w844 -> [w1857]
      tunnel: w843 -> [_]
      tunnel: w840 -> [w1853]
      tunnel: w839 -> [w1852]
      tunnel: w838 -> [w1849]
      tunnel: w837 -> [w1848]
      tunnel: w836 -> [w1847]
      tunnel: w835 -> [w1846]
      tunnel: w834 -> [_]
      tunnel: w833 -> [_]
      tunnel: [w1810] -> w832
      tunnel: [w1812] -> w831
      tunnel: [w1827] -> w828
      tunnel: [w1830] -> w827
      tunnel: [w1829] -> w826
      tunnel: w822 -> [w1844]
      tunnel: w821 -> [w1842]
      tunnel: w820 -> [w1840]
      tunnel: w819 -> [w1839]
      tunnel: w818 -> [w1838]
      tunnel: w817 -> [w1837]
      tunnel: w816 -> [w1836]
      tunnel: w815 -> [w1835]
      tunnel: w814 -> [w1834]
      tunnel: w813 -> [_]
      tunnel: w812 -> [_]
      tunnel: w811 -> [_]
      tunnel: [w1815] -> w810
      tunnel: [w1813] -> w809
      tunnel: [w1802] -> w808
      tunnel: [w1803] -> w807
      tunnel: [w1793] -> w663
      tunnel: [w1795] -> w615
      tunnel: w614 -> [w1799]
      tunnel: w613 -> [w1798]
      tunnel: w612 -> [_]
      tunnel: [w1796] -> w610
      tunnel: w607 -> [w1790]
      tunnel: w604 -> [w1785]
      tunnel: w603 -> [w1782]
      tunnel: w602 -> [w1780]
      tunnel: w601 -> [w1763]
      tunnel: w597 -> [w1779]
      tunnel: w596 -> [w1778]
      tunnel: [w1777] -> w595
      tunnel: w594 -> [w1776]
      tunnel: [w1775] -> w593
      tunnel: w592 -> [w1774]
      tunnel: w591 -> [w1773]
      tunnel: w590 -> [w1772]
      tunnel: w589 -> [w1771]
      tunnel: [w1770] -> w588
      tunnel: [w1769] -> w587
      tunnel: w586 -> [w1768]
      tunnel: [w1767] -> w569
      tunnel: [w1766] -> w567
      tunnel: [w1765] -> w577
      tunnel: w584 -> [w1757]
      tunnel: w583 -> [w1761]
      tunnel: w582 -> [w1760]
      tunnel: [w1759] -> w581
      tunnel: w558 -> [w1752]
      tunnel: w557 -> [w1755]
      tunnel: w556 -> [w1754]
      tunnel: w555 -> [w1753]
      tunnel: w554 -> [w1747]
      tunnel: w553 -> [w1750]
      tunnel: w551 -> [w1732]
      tunnel: w550 -> [w1746]
      tunnel: w549 -> [w1745]
      tunnel: [w1738] -> w548
      tunnel: [w1737] -> w547
      tunnel: [w1736] -> w546
      tunnel: [w1735] -> w545
      tunnel: w532 -> [w1711]
      tunnel: w531 -> [w1730]
      tunnel: w530 -> [w1729]
      tunnel: [w1728] -> w529
      tunnel: w490 -> [w1713]
      tunnel: w489 -> [w1712]
      tunnel: w486 -> [w1707]
      tunnel: w485 -> [w1709]
      tunnel: w484 -> [w1708]
      tunnel: w483 -> [w1705]
      tunnel: [w1702] -> w482
      tunnel: [w1701] -> w481
      frame #0 {
        # "Read and Resolve Data."
        # "Read/Resolve Symbol N"
        # "Read Data and Resolve Type"
        n266 = call-poly <userlib>:"Read TypeResolved.vi"("Handle"=w1573, "SymbolName"=w1644, "error constant"=w1582) -> ("Handle"=w1637:u32, "Read Status?"=w1642:bool, "RData"=w1638:variant, "error out"=w1641:errorcluster)  [unwired: 9 in]
        n267 = call-poly <userlib>:"Read TypeResolved.vi"("Handle"=w1573, "SymbolName"=w1645, "error constant"=w1582) -> ("Handle"=w1636:u32, "Read Status?"=w1643:bool, "RData"=w1639:variant, "error out"=w1640:errorcluster)  [unwired: 9 in]
        n268 = call-poly <userlib>:"Read TypeResolved.vi"("Handle"=w1573, "SymbolName"=w1698, "error constant"=w1582) -> ("Handle"=w1688:u32, "Read Status?"=w1690:bool, "RData"=w1694:variant, "error out"=w1699:errorcluster)  [unwired: 9 in]
        n269 = call-poly <userlib>:"Read TypeResolved.vi"("Handle"=w1573, "SymbolName"=w1649, "error constant"=w1582) -> ("Handle"=w1646:u32, "Read Status?"=w1648:bool, "RData"=w1647:variant, "error out"=w1651:errorcluster)  [unwired: 9 in]
        n270 = call-poly <userlib>:"Read TypeResolved.vi"("Handle"=w1573, "SymbolName"=w1700, "error constant"=w1582) -> ("Handle"=w1687:u32, "Read Status?"=w1689:bool, "RData"=w1693:variant, "error out"=w1650:errorcluster)  [unwired: 9 in]
        n271 = call-poly <userlib>:"Read TypeResolved.vi"("Handle"=w1573, "SymbolName"=w1576) -> ("Read Status?"=w1575:bool, "RData"=w1578:variant, "error out"=w1577:errorcluster)  [unwired: 10 in, 1 out]
        n272 = call-poly <userlib>:"Read TypeResolved.vi"("Handle"=w1573, "SymbolName"=w1696) -> ("Handle"=w1695:u32, "Read Status?"=w1691:bool, "RData"=w1692:variant, "error out"=w1697:errorcluster)  [unwired: 10 in]
        n273 = call-poly <userlib>:"Read TypeResolved.vi"("Handle"=w1573, "SymbolName"=w1686, "error constant"=w1582) -> ("Handle"=w1668:u32, "Read Status?"=w1675:bool, "RData"=w1667:variant, "error out"=w1674:errorcluster)  [unwired: 9 in]
        n274 = call-poly <userlib>:"Read TypeResolved.vi"("Handle"=w1573, "SymbolName"=w1587, "error constant"=w1582) -> ("Read Status?"=w1586:bool, "RData"=w1585:variant, "error out"=w1584:errorcluster)  [unwired: 9 in, 1 out]
        n275 = call-poly <userlib>:"Read TypeResolved.vi"("Handle"=w1573, "SymbolName"=w1574) -> ("Read Status?"=w1571:bool, "RData"=w1570:variant, "error out"=w1572:errorcluster)  [unwired: 10 in, 1 out]
        n276 = call-poly <userlib>:"Read TypeResolved.vi"("Handle"=w1573, "SymbolName"=w1583, "error constant"=w1582) -> ("Read Status?"=w1581:bool, "RData"=w1579:variant, "error out"=w1580:errorcluster)  [unwired: 9 in, 1 out]
        n277 = call-poly <userlib>:"Read TypeResolved.vi"("Handle"=w1573, "SymbolName"=w1684, "error constant"=w1582) -> ("Handle"=w1664:u32, "Read Status?"=w1677:bool, "RData"=w1663:variant, "error out"=w1672:errorcluster)  [unwired: 9 in]
        n278 = call-poly <userlib>:"Read TypeResolved.vi"("Handle"=w1573, "SymbolName"=w1682, "error constant"=w1582) -> ("Handle"=w1660:u32, "Read Status?"=w1679:bool, "RData"=w1659:variant, "error out"=w1670:errorcluster)  [unwired: 9 in]
        n279 = call-poly <userlib>:"Read TypeResolved.vi"("Handle"=w1573, "SymbolName"=w1599, "error constant"=w1582) -> ("Read Status?"=w1598:bool, "RData"=w1597:variant, "error out"=w1596:errorcluster)  [unwired: 9 in, 1 out]
        n280 = call-poly <userlib>:"Read TypeResolved.vi"("Handle"=w1573, "SymbolName"=w1595, "error constant"=w1582) -> ("Read Status?"=w1593:bool, "RData"=w1592:variant, "error out"=w1591:errorcluster)  [unwired: 9 in, 1 out]
        n281 = call-poly <userlib>:"Read TypeResolved.vi"("Handle"=w1573, "SymbolName"=w1594, "error constant"=w1582) -> ("Read Status?"=w1589:bool, "RData"=w1588:variant, "error out"=w1590:errorcluster)  [unwired: 9 in, 1 out]
        n282 = call-poly <userlib>:"Read TypeResolved.vi"("Handle"=w1573, "SymbolName"=w1685, "error constant"=w1582) -> ("Handle"=w1666:u32, "Read Status?"=w1676:bool, "RData"=w1665:variant, "error out"=w1673:errorcluster)  [unwired: 9 in]
        n283 = call-poly <userlib>:"Read TypeResolved.vi"("Handle"=w1573, "SymbolName"=w1683, "error constant"=w1582) -> ("Handle"=w1662:u32, "Read Status?"=w1678:bool, "RData"=w1661:variant, "error out"=w1671:errorcluster)  [unwired: 9 in]
        n284 = call-poly <userlib>:"Read TypeResolved.vi"("Handle"=w1573, "SymbolName"=w1681, "error constant"=w1582) -> ("Handle"=w1658:u32, "Read Status?"=w1680:bool, "RData"=w1657:variant, "error out"=w1669:errorcluster)  [unwired: 9 in]
        n285 = call-poly <userlib>:"Read TypeResolved.vi"("Handle"=w1573, "SymbolName"=w1656, "error constant"=w1582) -> ("Handle"=w1653:u32, "Read Status?"=w1652:bool, "RData"=w1655:variant, "error out"=w1654:errorcluster)  [unwired: 9 in]
        n286 = call-poly <userlib>:"Read TypeResolved.vi"("Handle"=w1573, "SymbolName"=w1615, "error constant"=w1582) -> ("Read Status?"=w1614:bool, "RData"=w1607:variant, "error out"=w1606:errorcluster)  [unwired: 9 in, 1 out]
        n287 = call-poly <userlib>:"Read TypeResolved.vi"("Handle"=w1573, "SymbolName"=w1610, "error constant"=w1582) -> ("Read Status?"=w1613:bool, "RData"=w1600:variant, "error out"=w1605:errorcluster)  [unwired: 9 in, 1 out]
        n288 = call-poly <userlib>:"Read TypeResolved.vi"("Handle"=w1573, "SymbolName"=w1608, "error constant"=w1582) -> ("Read Status?"=w1611:bool, "RData"=w1601:variant, "error out"=w1602:errorcluster)  [unwired: 9 in, 1 out]
        n289 = call-poly <userlib>:"Read TypeResolved.vi"("Handle"=w1573, "SymbolName"=w1609, "error constant"=w1582) -> ("Read Status?"=w1612:bool, "RData"=w1603:variant, "error out"=w1604:errorcluster)  [unwired: 9 in, 1 out]
        n290 = call-poly <userlib>:"Read TypeResolved.vi"("Handle"=w1573, "SymbolName"=w1635, "error constant"=w1582) -> ("Handle"=w1623:u32, "Read Status?"=w1632:bool, "RData"=w1628:variant, "error out"=w1624:errorcluster)  [unwired: 9 in]
        n291 = call-poly <userlib>:"Read TypeResolved.vi"("Handle"=w1573, "SymbolName"=w1634, "error constant"=w1582) -> ("Handle"=w1622:u32, "Read Status?"=w1631:bool, "RData"=w1629:variant, "error out"=w1625:errorcluster)  [unwired: 9 in]
        n292 = call-poly <userlib>:"Read TypeResolved.vi"("Handle"=w1573, "SymbolName"=w1617, "error constant"=w1582) -> ("Handle"=w1618:u32, "Read Status?"=w1616:bool, "RData"=w1620:variant, "error out"=w1619:errorcluster)  [unwired: 9 in]
        n293 = call-poly <userlib>:"Read TypeResolved.vi"("Handle"=w1573, "SymbolName"=w1633, "error constant"=w1582) -> ("Handle"=w1621:u32, "Read Status?"=w1630:bool, "RData"=w1627:variant, "error out"=w1626:errorcluster)  [unwired: 9 in]
      }
      frame #1 {
        # "Cast Symbol N to LabVIEW Type"
        # "Variant To Data"
        n294 = And(x=w1707, y=w1708) -> (x .and. y?=w1706:bool)
        n295 = And(x=w1711, y=w1706) -> (x .and. y?=w1710:bool)
        n296 = Variant To Data(error in=w1712, Variant=w1713) -> (data=→"Test Interval (Sec)":i32, error out=w1702:errorcluster)  [unwired: 1 in]
        n297 = Variant To Data(error in=w1709, Variant=w1705) -> (data=→"Test Interval Fault":bool, error out=w1701:errorcluster)  [unwired: 1 in]
        n298 = And(x=w1732, y=w1710) -> (x .and. y?=w1731:bool)
        n299 = And(x=w1747, y=w1731) -> (x .and. y?=w1748:bool)
        n300 = And(x=w1752, y=w1748) -> (x .and. y?=w1751:bool)
        n301 = And(x=w1757, y=w1751) -> (x .and. y?=w1756:bool)
        n302 = And(x=w1763, y=w1756) -> (x .and. y?=w1762:bool)
        n303 = And(x=w1780, y=w1762) -> (x .and. y?=w1781:bool)
        n304 = And(x=w1782, y=w1781) -> (x .and. y?=w1783:bool)
        n305 = And(x=w1785, y=w1783) -> (x .and. y?=w1784:bool)
        n306 = And(x=w1787, y=w1784) -> (x .and. y?=w1786:bool)
        n307 = And(x=w1884, y=w1786) -> (x .and. y?=w1900:bool)
        n308 = And(x=w1899, y=w1900) -> (x .and. y?=w1898:bool)
        n309 = And(x=w1897, y=w1898) -> (x .and. y?=w1896:bool)
        n310 = And(x=w1895, y=w1896) -> (x .and. y?=w1894:bool)
        n311 = And(x=w1893, y=w1894) -> (x .and. y?=w1892:bool)
        n312 = And(x=w1891, y=w1892) -> (x .and. y?=w1890:bool)
        n313 = And(x=w1901, y=w1890) -> (x .and. y?=w1845:bool)
        n314 = And(x=w1844, y=w1845) -> (x .and. y?=w1843:bool)
        n315 = And(x=w1842, y=w1843) -> (x .and. y?=w1841:bool)
        n316 = And(x=w1840, y=w1841) -> (x .and. y?=w1789:bool)
        n317 = And(x=w1790, y=w1789) -> (x .and. y?=w1788:bool)
        n318 = And(x=w1852, y=w1788) -> (x .and. y?=w1851:bool)
        n319 = And(x=w1853, y=w1851) -> (x .and. y?=w1850:bool)
        n320 = And(x=w1859, y=w1850) -> (x .and. y?=w1858:bool)
        n321 = And(x=w1906, y=w1858) -> (x .and. y?=w1905:bool)
        n322 = Variant To Data(error in=w1798, Variant=w1799) -> (data=→"Cap 1 Voltage (HVPS)":i16, error out=w1796:errorcluster)  [unwired: 1 in]
        n323 = Variant To Data(error in=w1883, Variant=w1877) -> (data=→"Discharge Fault":bool, error out=w1819:errorcluster)  [unwired: 1 in]
        n324 = Variant To Data(error in=w1902, Variant=w1903) -> (data=→"Charge Fault":bool, error out=w1817:errorcluster)  [unwired: 1 in]
        n325 = Variant To Data(error in=w1881, Variant=w1875) -> (data=→"Cap 1 Temp\nExceeded Fault":bool, error out=w1823:errorcluster)  [unwired: 1 in]
        n326 = And(x=w1904, y=w1905) -> (x .and. y?=→"Read Status":bool)
        n327 = Variant To Data(error in=w1882, Variant=w1876) -> (data=→"Hold Fault":bool, error out=w1821:errorcluster)  [unwired: 1 in]
        n328 = Variant To Data(error in=w1836, Variant=w1837) -> (data=→"Load Temperature":i16, error out=w1802:errorcluster)  [unwired: 1 in]
        n329 = Variant To Data(error in=w1880, Variant=w1874) -> (data=→"Ambient Temp\nExceeded Fault":bool, error out=w1825:errorcluster)  [unwired: 1 in]
        n330 = Variant To Data(error in=w1879, Variant=w1873) -> (data=→"PSU Fault":bool, error out=w1827:errorcluster)  [unwired: 1 in]
        n331 = Variant To Data(error in=w1878, Variant=w1872) -> (data=→"Control Sys Fault":bool, error out=w1829:errorcluster)  [unwired: 1 in]
        n332 = Variant To Data(error in=w1861, Variant=w1862) -> (data=→"test Running":bool, error out=w1830:errorcluster)  [unwired: 1 in]
        n333 = Variant To Data(error in=w1834, Variant=w1838) -> (data=→"Ambient Temp":i16, error out=w1815:errorcluster)  [unwired: 1 in]
        n334 = Variant To Data(error in=w1772, Variant=w1771) -> (data=w1765:bool, error out=w1769:errorcluster)  [unwired: 1 in]
        "Soft Exception" <- w1765
        n335 = Variant To Data(error in=w1760, Variant=w1761) -> (data=w1758:bool, error out=w1738:errorcluster)  [unwired: 1 in]
        "EOC" <- w1758
        n336 = Variant To Data(error in=w1835, Variant=w1839) -> (data=→"Soft Dump Temp":i16, error out=w1813:errorcluster)  [unwired: 1 in]
        n337 = Variant To Data(error in=w1778, Variant=w1779) -> (data=w1759:bool, error out=w1777:errorcluster)  [unwired: 1 in]
        "Softdump FB Fault" <- w1759
        n338 = Variant To Data(error in=w1774, Variant=w1773) -> (data=w1766:bool, error out=w1770:errorcluster)  [unwired: 1 in]
        "PSU HV FB Fault" <- w1766
        n339 = Variant To Data(error in=w1754, Variant=w1755) -> (data=w1725:bool, error out=w1737:errorcluster)  [unwired: 1 in]
        "SCR Ready" <- w1725
        n340 = Variant To Data(error in=w1753, Variant=w1750) -> (data=→"Maximum Test Number Reached":bool, error out=w1736:errorcluster)  [unwired: 1 in]
        n341 = Variant To Data(error in=w1776, Variant=w1768) -> (data=w1767:bool, error out=w1775:errorcluster)  [unwired: 1 in]
        "Charge FB Fault" <- w1767
        n342 = Variant To Data(error in=w1730, Variant=w1729) -> (data=w1726:bool, error out=w1728:errorcluster)  [unwired: 1 in]
        "Scope Trig" <- w1726
        n343 = Variant To Data(error in=w1856, type=2, Variant=w1857) -> (data=w1727:i32, error out=w1808:errorcluster)
        "Process Step" <- w1727
        n344 = Variant To Data(error in=w1849, Variant=w1846) -> (data=→"Cap 1 Temperature":i16, error out=w1812:errorcluster)  [unwired: 1 in]
        n345 = Variant To Data(error in=w1848, Variant=w1847) -> (data=w1744:i16, error out=w1810:errorcluster)  [unwired: 1 in]
        "Cap 1 Voltage" <- w1744
        n346 = Variant To Data(error in=w1745, Variant=w1746) -> (data=w1734:i16, error out=w1735:errorcluster)  [unwired: 1 in]
        "Expected Voltage" <- w1734
        n347 = Variant To Data(error in=w1889, Variant=w1888) -> (data=→"Estimated Charge Time (seconds)":sgl, error out=w1804:errorcluster)  [unwired: 1 in]
        n348 = To Double Precision Float(number=w1744) -> (double precision float=→"Waveform Chart - Capacitor Voltage (Probe, abs(Volts))":dbl)
        n349 = Variant To Data(error in=w1860, Variant=w1887) -> (data=→"Shot Number":i32, error out=w1806:errorcluster)  [unwired: 1 in]
        n350 = case shown="True" "Log Temperature Data" {
          tunnel: [errorcluster {"status"=FALSE, "code"=0, "source"=""} ("error out") w1916] -> w1795
          frame False {
          }
          frame True {
            n351 = local read "Cap 1 Temperature"() -> (w1917:i16)
            n352 = local read "test Running"() -> (w1915:bool)
            n353 = call "Write To Measurement File2"("Signals"=w1917, "Enable"=w1915, "Filename"="Capacitor Temperature Data Log File Path (.xlsx)") -> ("error out"=w1916:errorcluster)  [unwired: 14 in, 2 out]
          }
        }
        n354 = case shown="5" w1727 {
          tunnel: ["Charge" "Current Controlled Charge" "Hold - Ready for Shot" "Hold - Cap Open Circuited" "Shot" "Wait" "Dump" "Error" "Wait"] -> w1855
          tunnel: [TRUE TRUE TRUE TRUE TRUE TRUE FALSE FALSE FALSE] -> w1723
          tunnel: [FALSE ("Reset") FALSE ("Reset") FALSE ("Reset") FALSE ("Reset") TRUE ("Reset") FALSE ("Reset") FALSE ("Reset") TRUE ("Reset") FALSE ("Reset")] -> _
          frame 1 {
          }
          frame 6 {
          }
          frame 2 {
          }
          frame 7 {
          }
          frame 3 {
          }
          frame 4 {
          }
          frame 5 {
          }
          frame 999 {
          }
          frame 0, Default {
          }
        }
        "Test State" <- w1855
        n355 = local write "Scope Trig"(w1726) -> ()
        n356 = local read "Cap 1 Voltage"() -> (w1715:i16)
        n357 = case shown="True" "Log Capacitor Voltage" {
          tunnel: [errorcluster {"status"=FALSE, "code"=0, "source"=""} ("error out") w1913] -> w1793
          tunnel: w1744 -> [_ w1912]
          tunnel: w1723 -> [_ w1911]
          frame False {
          }
          frame True {
            n358 = local read "test Running"() -> (w1908:bool)
            n359 = And(x=w1911, y=w1908) -> (x .and. y?=w1909:bool)
            n360 = call "Write To Measurement File"("Signals"=w1912, "Enable"=w1909, "Filename"="Capacitor Voltage Data Log File Path (.xlsx)") -> ("error out"=w1913:errorcluster)  [unwired: 14 in, 2 out]
          }
        }
        n361 = Not(x=w1758) -> (.not. x?=w1742:bool)
        n362 = To Double Precision Float(number=w1715) -> (double precision float=w1740:dbl)
        n363 = To Double Precision Float(number=w1734) -> (double precision float=w1733:dbl)
        n364 = Boolean To (0,1)(Boolean=w1742) -> (0, 1=→"EOC":i16)
        n365 = Or(x=w1829, y=w1830) -> (x .or. y?=w1828:bool)
        n366 = Or(x=w1827, y=w1828) -> (x .or. y?=w1826:bool)
        n367 = Or(x=w1825, y=w1826) -> (x .or. y?=w1824:bool)
        n368 = Or(x=w1823, y=w1824) -> (x .or. y?=w1822:bool)
        n369 = Or(x=w1821, y=w1822) -> (x .or. y?=w1820:bool)
        n370 = Or(x=w1819, y=w1820) -> (x .or. y?=w1818:bool)
        n371 = Or(x=w1817, y=w1818) -> (x .or. y?=w1816:bool)
        n372 = Or(x=w1815, y=w1816) -> (x .or. y?=w1814:bool)
        n373 = Or(x=w1813, y=w1814) -> (x .or. y?=w1801:bool)
        n374 = Or(x=w1802, y=w1801) -> (x .or. y?=w1794:bool)
        n375 = Boolean To (0,1)(Boolean=w1725) -> (0, 1=→"SCR FB":i16)
        n376 = Bundle(w1740, w1733) -> (→"Capacitor Voltage":cluster{dbl, dbl})  [unwired: 1 in]
        n377 = local read "Scope Trig"() -> (w1718:bool)
        n378 = local write "Process Step"(w1727) -> ()
        n379 = Not(x=w1718) -> (.not. x?=w1717:bool)
        n380 = local read "Test Interval (Sec)"() -> (w1721:i32)
        n381 = call "Elapsed Time"("Time Target (s)"=w1721, "Reset"=w1717) -> ("Elapsed Time Text"=w1720:string)  [unwired: 10 in, 7 out]
        n382 = String Subset(string=w1720, offset (0)=2) -> (substring=→"Time Since Last Shot":string)  [unwired: 1 in]
        n383 = Or(x=w1795, y=w1794) -> (x .or. y?=w1792:bool)
        n384 = Or(x=w1793, y=w1792) -> (x .or. y?=w1791:bool)
        n385 = Or(x=w1812, y=w1791) -> (x .or. y?=w1811:bool)
        n386 = Or(x=w1810, y=w1811) -> (x .or. y?=w1809:bool)
        n387 = Or(x=w1808, y=w1809) -> (x .or. y?=w1807:bool)
        n388 = Or(x=w1806, y=w1807) -> (x .or. y?=w1805:bool)
        n389 = Or(x=w1804, y=w1805) -> (x .or. y?=w1803:bool)
        "Internal TwinCAT Handle ID Maps" <- w1864
      }
    }
    n390 = call-poly <userlib>:"Write TypeResolved.vi"("Handle"=w506, "SymbolName"=w544, "WData"=w536, "error constant"=w543) -> ("Handle"=w537:u32, "Write Status?"=w492:bool, "Has Matched?"=w500:bool, "error out"=w538:errorcluster)  [unwired: 8 in]
    n391 = call <userlib>:"Send Writer-Request.vi"("Handle"=w801, "SymbolName"=w800, "WriterMode"=w799, "WriteHandle"=w797, "error constant"=w798, "ADS Write Data"=w796) -> ("Handle"=w792:u32, "WriteHandle"=w791:u32, "Write status?"=w618:bool, "error IO"=w666:errorcluster)  [unwired: 5 in, 1 out]
    n392 = call <userlib>:"Send Writer-Request.vi"("Handle"=w634, "SymbolName"=w633, "WriterMode"=w632, "WriteHandle"=w631, "error constant"=w630, "ADS Write Data"=w626) -> ("Handle"=w625:u32, "WriteHandle"=w622:u32, "Write status?"=w542:bool, "error IO"=w617:errorcluster)  [unwired: 5 in, 1 out]
    n393 = call <userlib>:"Send Writer-Request.vi"("Handle"=w972, "SymbolName"=w971, "WriterMode"=w970, "WriteHandle"=w968, "error constant"=w969, "ADS Write Data"=w879) -> ("Handle"=w967:u32, "WriteHandle"=w966:u32, "Write status?"=w518:bool, "error IO"=w687:errorcluster)  [unwired: 5 in, 1 out]
    n394 = call <userlib>:"Send Writer-Request.vi"("Handle"=w912, "SymbolName"=w911, "WriterMode"=w910, "WriteHandle"=w909, "error constant"=w908, "ADS Write Data"=w874) -> ("Handle"=w904:u32, "WriteHandle"=w903:u32, "Write status?"=w513:bool, "error IO"=w672:errorcluster)  [unwired: 5 in, 1 out]
    n395 = call <userlib>:"Send Writer-Request.vi"("Handle"=w868, "SymbolName"=w867, "WriterMode"=w866, "WriteHandle"=w857, "error constant"=w865, "ADS Write Data"=w869) -> ("Handle"=w864:u32, "WriteHandle"=w863:u32, "Write status?"=w512:bool, "error IO"=w669:errorcluster)  [unwired: 5 in, 1 out]
    n396 = call <userlib>:"Send Writer-Request.vi"("Handle"=w960, "SymbolName"=w959, "WriterMode"=w958, "WriteHandle"=w957, "error constant"=w956, "ADS Write Data"=w878) -> ("Handle"=w952:u32, "WriteHandle"=w951:u32, "Write status?"=w517:bool, "error IO"=w684:errorcluster)  [unwired: 5 in, 1 out]
    n397 = call <userlib>:"Send Writer-Request.vi"("Handle"=w936, "SymbolName"=w935, "WriterMode"=w934, "WriteHandle"=w933, "error constant"=w932, "ADS Write Data"=w876) -> ("Handle"=w928:u32, "WriteHandle"=w927:u32, "Write status?"=w515:bool, "error IO"=w678:errorcluster)  [unwired: 5 in, 1 out]
    n398 = call <userlib>:"Send Writer-Request.vi"("Handle"=w948, "SymbolName"=w947, "WriterMode"=w946, "WriteHandle"=w945, "error constant"=w944, "ADS Write Data"=w877) -> ("Handle"=w940:u32, "WriteHandle"=w939:u32, "Write status?"=w516:bool, "error IO"=w681:errorcluster)  [unwired: 5 in, 1 out]
    n399 = call <userlib>:"Send Writer-Request.vi"("Handle"=w924, "SymbolName"=w923, "WriterMode"=w922, "WriteHandle"=w921, "error constant"=w920, "ADS Write Data"=w875) -> ("Handle"=w916:u32, "WriteHandle"=w915:u32, "Write status?"=w514:bool, "error IO"=w675:errorcluster)  [unwired: 5 in, 1 out]
    n400 = call <userlib>:"Send Writer-Request.vi"("Handle"=w1044, "SymbolName"=w1043, "WriterMode"=w1042, "WriteHandle"=w1040, "error constant"=w1041, "ADS Write Data"=w885) -> ("Handle"=w1039:u32, "WriteHandle"=w1038:u32, "Write status?"=w741:bool, "error IO"=w704:errorcluster)  [unwired: 5 in, 1 out]
    n401 = call <userlib>:"Send Writer-Request.vi"("Handle"=w984, "SymbolName"=w983, "WriterMode"=w982, "WriteHandle"=w981, "error constant"=w980, "ADS Write Data"=w880) -> ("Handle"=w976:u32, "WriteHandle"=w975:u32, "Write status?"=w751:bool, "error IO"=w689:errorcluster)  [unwired: 5 in, 1 out]
    n402 = call <userlib>:"Send Writer-Request.vi"("Handle"=w1032, "SymbolName"=w1031, "WriterMode"=w1030, "WriteHandle"=w1029, "error constant"=w1028, "ADS Write Data"=w884) -> ("Handle"=w1024:u32, "WriteHandle"=w1023:u32, "Write status?"=w743:bool, "error IO"=w701:errorcluster)  [unwired: 5 in, 1 out]
    n403 = call <userlib>:"Send Writer-Request.vi"("Handle"=w1008, "SymbolName"=w1007, "WriterMode"=w1006, "WriteHandle"=w1005, "error constant"=w1004, "ADS Write Data"=w882) -> ("Handle"=w1000:u32, "WriteHandle"=w999:u32, "Write status?"=w747:bool, "error IO"=w695:errorcluster)  [unwired: 5 in, 1 out]
    n404 = call <userlib>:"Send Writer-Request.vi"("Handle"=w1020, "SymbolName"=w1019, "WriterMode"=w1018, "WriteHandle"=w1017, "error constant"=w1016, "ADS Write Data"=w883) -> ("Handle"=w1012:u32, "WriteHandle"=w1011:u32, "Write status?"=w745:bool, "error IO"=w698:errorcluster)  [unwired: 5 in, 1 out]
    n405 = call <userlib>:"Send Writer-Request.vi"("Handle"=w996, "SymbolName"=w995, "WriterMode"=w994, "WriteHandle"=w993, "error constant"=w992, "ADS Write Data"=w881) -> ("Handle"=w988:u32, "WriteHandle"=w987:u32, "Write status?"=w749:bool, "error IO"=w692:errorcluster)  [unwired: 5 in, 1 out]
    n406 = call <userlib>:"Send Writer-Request.vi"("Handle"=w658, "SymbolName"=w657, "WriterMode"=w656, "WriteHandle"=w655, "error constant"=w654, "ADS Write Data"=w650) -> ("Handle"=w649:u32, "WriteHandle"=w648:u32, "Write status?"=w642:bool, "error IO"=w641:errorcluster)  [unwired: 5 in, 1 out]
    n407 = Compound Arithmetic op=AND(w500, w498, w497, w496) -> (w499:bool)
    n408 = And(x=w540, y=w499) -> (x .and. y?=w539:bool)
    n409 = And(x=w621, y=w539) -> (x .and. y?=w620:bool)
    n410 = And(x=w737, y=w620) -> (x .and. y?=w736:bool)
    n411 = And(x=w735, y=w736) -> (x .and. y?=w734:bool)
    n412 = And(x=w733, y=w734) -> (x .and. y?=w732:bool)
    n413 = And(x=w731, y=w732) -> (x .and. y?=w730:bool)
    n414 = And(x=w729, y=w730) -> (x .and. y?=w728:bool)
    n415 = And(x=w727, y=w728) -> (x .and. y?=w726:bool)
    n416 = And(x=w725, y=w726) -> (x .and. y?=w609:bool)
    n417 = And(x=w644, y=w609) -> (x .and. y?=w645:bool)
    n418 = And(x=w724, y=w645) -> (x .and. y?=w723:bool)
    n419 = And(x=w722, y=w723) -> (x .and. y?=w721:bool)
    n420 = And(x=w720, y=w721) -> (x .and. y?=w719:bool)
    n421 = And(x=w718, y=w719) -> (x .and. y?=w717:bool)
    n422 = And(x=w716, y=w717) -> (x .and. y?=w715:bool)
    n423 = And(x=w714, y=w715) -> (x .and. y?=w713:bool)
    n424 = And(x=w712, y=w713) -> (x .and. y?=w711:bool)
    n425 = And(x=w739, y=w711) -> (x .and. y?=→"bHasMached":bool)
    n426 = Compound Arithmetic op=AND(w492, w493, w494, w495) -> (w491:bool)
    n427 = And(x=w542, y=w491) -> (x .and. y?=w541:bool)
    n428 = And(x=w618, y=w541) -> (x .and. y?=w509:bool)
    n429 = Compound Arithmetic op=AND(w518, w517, w516, w515, w514, w513, w512) -> (w511:bool)
    n430 = Not(x=w511) -> (.not. x?=w510:bool)
    n431 = And(x=w510, y=w509) -> (x .and. y?=w508:bool)
    n432 = And(x=w642, y=w508) -> (x .and. y?=w643:bool)
    n433 = And(x=w751, y=w643) -> (x .and. y?=w750:bool)
    n434 = And(x=w749, y=w750) -> (x .and. y?=w748:bool)
    n435 = And(x=w747, y=w748) -> (x .and. y?=w746:bool)
    n436 = And(x=w745, y=w746) -> (x .and. y?=w744:bool)
    n437 = And(x=w743, y=w744) -> (x .and. y?=w742:bool)
    n438 = And(x=w741, y=w742) -> (x .and. y?=w740:bool)
    n439 = And(x=w753, y=w740) -> (x .and. y?=w752:bool)
    n440 = And(x=w754, y=w752) -> (x .and. y?=→"Write Status":bool)
    n441 = feedback #2(TRUE) -> (w564:bool)
    n442 = And(x=w564, y=w567) -> (x .and. y?=w566:bool)
    n443 = feedback #3(TRUE) -> (w574:bool)
    n444 = And(x=w574, y=w577) -> (x .and. y?=w576:bool)
    n445 = feedback #4(TRUE) -> (w578:bool)
    n446 = And(x=w578, y=w581) -> (x .and. y?=w580:bool)
    n447 = feedback #5(TRUE) -> (w570:bool)
    n448 = And(x=w570, y=w569) -> (x .and. y?=w571:bool)
    n449 = case shown="True" w571 {
      tunnel: [w1255 FALSE] -> w561
      tunnel: w562 -> [w1257 _]
      frame False {
        n450 = Or(x=w1257, y=FALSE) -> (x .or. y?=w1255:bool)
      }
      frame True {
        n451 = call "Charge relay error"() -> ()  [unwired: 10 in, 2 out]
      }
    }
    n452 = feedback-in #5(w561) -> ()
    n453 = case shown="True" w566 {
      tunnel: [w1253 FALSE] -> w565
      tunnel: w561 -> [w1251 _]
      frame False {
        n454 = Or(x=w1251, y=FALSE) -> (x .or. y?=w1253:bool)
      }
      frame True {
        n455 = call "PSU HV error"() -> ()  [unwired: 10 in, 2 out]
      }
    }
    n456 = feedback-in #2(w565) -> ()
    n457 = case shown="True" w580 {
      tunnel: [w1264 FALSE] -> w579
      tunnel: w562 -> [w1263 _]
      frame False {
        n458 = Or(x=w1263, y=FALSE) -> (x .or. y?=w1264:bool)
      }
      frame True {
        n459 = call "Softdump error"() -> ()  [unwired: 10 in, 2 out]
      }
    }
    n460 = feedback-in #4(w579) -> ()
    n461 = case shown="True" w576 {
      tunnel: [w1259 FALSE] -> w575
      tunnel: w561 -> [w1260 _]
      frame False {
        n462 = Or(x=w1260, y=FALSE) -> (x .or. y?=w1259:bool)
      }
      frame True {
        n463 = call "Soft Exception"() -> ()  [unwired: 10 in, 2 out]
      }
    }
    n464 = feedback-in #3(w575) -> ()
    n465 = Compound Arithmetic op=OR(w664, w710, w709) -> (w708:bool)
    n466 = Compound Arithmetic op=OR(w708, w707, w706) -> (w705:bool)
    n467 = Compound Arithmetic op=OR(w705, w704, w703) -> (w702:bool)
    n468 = Compound Arithmetic op=OR(w702, w701, w700) -> (w699:bool)
    n469 = Compound Arithmetic op=OR(w699, w698, w697) -> (w696:bool)
    n470 = Compound Arithmetic op=OR(w696, w695, w694) -> (w693:bool)
    n471 = Compound Arithmetic op=OR(w693, w692, w691) -> (w690:bool)
    n472 = Compound Arithmetic op=OR(w690, w689, w688) -> (w639:bool)
    n473 = Compound Arithmetic op=OR(w639, w641, w640) -> (w608:bool)
    n474 = Compound Arithmetic op=OR(w608, w687, w686) -> (w685:bool)
    n475 = Compound Arithmetic op=OR(w685, w684, w683) -> (w682:bool)
    n476 = Compound Arithmetic op=OR(w682, w681, w680) -> (w679:bool)
    n477 = Compound Arithmetic op=OR(w679, w678, w677) -> (w676:bool)
    n478 = Compound Arithmetic op=OR(w676, w675, w674) -> (w673:bool)
    n479 = Compound Arithmetic op=OR(w673, w672, w671) -> (w670:bool)
    n480 = Compound Arithmetic op=OR(w670, w669, w668) -> (w667:bool)
    n481 = Compound Arithmetic op=OR(w667, w666, w665) -> (w619:bool)
    n482 = Compound Arithmetic op=OR(w619, w617, w616) -> (w480:bool)
    n483 = Compound Arithmetic op=OR(w480, "EXIT HMI", w807) -> (w606:bool)
    "Stop Loops" <- w606
    n484 = property on="Stop Loops" class="Bool (strict)"("Val(Sgnl)"=w606) -> ()  [unwired: 2 in, 2 out]
    n485 = node-c288() -> ()  [unwired: 1 in, 1 out]
  }
  n486 = node-c288(w103) -> (w101:errorcluster)
  n487 = call <userlib>:"Release Writer.vi"("Handle"=w217, "WriteHandle"=w216, "error in (no error)"=w215) -> ("error out"=w211:errorcluster)  [unwired: 11 in, 1 out]
  n488 = call <userlib>:"Release Writer.vi"("Handle"=w313, "WriteHandle"=w312, "error in (no error)"=w311) -> ("error out"=w319:errorcluster)  [unwired: 11 in, 1 out]
  n489 = call <userlib>:"Release Writer.vi"("Handle"=w293, "WriteHandle"=w292, "error in (no error)"=w291) -> ("error out"=w287:errorcluster)  [unwired: 11 in, 1 out]
  n490 = call <userlib>:"Release Writer.vi"("Handle"=w255, "WriteHandle"=w254, "error in (no error)"=w253) -> ("error out"=w249:errorcluster)  [unwired: 11 in, 1 out]
  n491 = call <userlib>:"Release Type.vi"("Handle"=w214, "TypeHandle"=w213, "error in (no error)"=w212) -> ("error out"=w210:errorcluster)  [unwired: 11 in, 1 out]
  n492 = call <userlib>:"Release Type.vi"("Handle"=w308, "TypeHandle"=w309, "error in (no error)"=w310) -> ("error out"=w320:errorcluster)  [unwired: 11 in, 1 out]
  n493 = call <userlib>:"Release Type.vi"("Handle"=w290, "TypeHandle"=w289, "error in (no error)"=w288) -> ("error out"=w286:errorcluster)  [unwired: 11 in, 1 out]
  n494 = call <userlib>:"Release Writer.vi"("Handle"=w274, "WriteHandle"=w273, "error in (no error)"=w272) -> ("error out"=w268:errorcluster)  [unwired: 11 in, 1 out]
  n495 = call <userlib>:"Release Type.vi"("Handle"=w252, "TypeHandle"=w251, "error in (no error)"=w250) -> ("error out"=w248:errorcluster)  [unwired: 11 in, 1 out]
  n496 = call <userlib>:"Release Writer.vi"("Handle"=w236, "WriteHandle"=w235, "error in (no error)"=w234) -> ("error out"=w230:errorcluster)  [unwired: 11 in, 1 out]
  n497 = call <userlib>:"Release Type.vi"("Handle"=w271, "TypeHandle"=w270, "error in (no error)"=w269) -> ("error out"=w267:errorcluster)  [unwired: 11 in, 1 out]
  n498 = call <userlib>:"Release Type.vi"("Handle"=w233, "TypeHandle"=w232, "error in (no error)"=w231) -> ("error out"=w229:errorcluster)  [unwired: 11 in, 1 out]
  n499 = call <userlib>:"Release Writer.vi"("Handle"=w462, "WriteHandle"=w461, "error in (no error)"=w473) -> ("error out"=w141:errorcluster)  [unwired: 11 in, 1 out]
  n500 = call <userlib>:"Release Writer.vi"("Handle"=w331, "WriteHandle"=w330, "error in (no error)"=w329) -> ("error out"=w325:errorcluster)  [unwired: 11 in, 1 out]
  n501 = call <userlib>:"Release Writer.vi"("Handle"=w427, "WriteHandle"=w426, "error in (no error)"=w425) -> ("error out"=w433:errorcluster)  [unwired: 11 in, 1 out]
  n502 = call <userlib>:"Release Writer.vi"("Handle"=w407, "WriteHandle"=w406, "error in (no error)"=w405) -> ("error out"=w401:errorcluster)  [unwired: 11 in, 1 out]
  n503 = call <userlib>:"Release Writer.vi"("Handle"=w369, "WriteHandle"=w368, "error in (no error)"=w367) -> ("error out"=w363:errorcluster)  [unwired: 11 in, 1 out]
  n504 = call <userlib>:"Release Type.vi"("Handle"=w328, "TypeHandle"=w327, "error in (no error)"=w326) -> ("error out"=w324:errorcluster)  [unwired: 11 in, 1 out]
  n505 = call <userlib>:"Release Type.vi"("Handle"=w422, "TypeHandle"=w423, "error in (no error)"=w424) -> ("error out"=w434:errorcluster)  [unwired: 11 in, 1 out]
  n506 = call <userlib>:"Release Type.vi"("Handle"=w404, "TypeHandle"=w403, "error in (no error)"=w402) -> ("error out"=w400:errorcluster)  [unwired: 11 in, 1 out]
  n507 = call <userlib>:"Release Writer.vi"("Handle"=w388, "WriteHandle"=w387, "error in (no error)"=w386) -> ("error out"=w382:errorcluster)  [unwired: 11 in, 1 out]
  n508 = call <userlib>:"Release Type.vi"("Handle"=w366, "TypeHandle"=w365, "error in (no error)"=w364) -> ("error out"=w362:errorcluster)  [unwired: 11 in, 1 out]
  n509 = call <userlib>:"Release Writer.vi"("Handle"=w350, "WriteHandle"=w349, "error in (no error)"=w348) -> ("error out"=w344:errorcluster)  [unwired: 11 in, 1 out]
  n510 = call <userlib>:"Release Type.vi"("Handle"=w385, "TypeHandle"=w384, "error in (no error)"=w383) -> ("error out"=w381:errorcluster)  [unwired: 11 in, 1 out]
  n511 = call <userlib>:"Release Type.vi"("Handle"=w347, "TypeHandle"=w346, "error in (no error)"=w345) -> ("error out"=w343:errorcluster)  [unwired: 11 in, 1 out]
  n512 = call <userlib>:"Release Writer.vi"("Handle"=w445, "WriteHandle"=w444, "error in (no error)"=w443) -> ("error out"=w439:errorcluster)  [unwired: 11 in, 1 out]
  n513 = call <userlib>:"Release Writer.vi"("Handle"=w85, "WriteHandle"=w84, "error in (no error)"=w83) -> ("error out"=w99:errorcluster)  [unwired: 11 in, 1 out]
  n514 = call <userlib>:"Release Writer.vi"("Handle"=w179, "WriteHandle"=w178, "error in (no error)"=w180) -> ("error out"=w186:errorcluster)  [unwired: 11 in, 1 out]
  n515 = call <userlib>:"Release Type.vi"("Handle"=w442, "TypeHandle"=w441, "error in (no error)"=w440) -> ("error out"=w438:errorcluster)  [unwired: 11 in, 1 out]
  n516 = call <userlib>:"Release Type.vi"("Handle"=w81, "TypeHandle"=w80, "error in (no error)"=w82) -> ("error out"=w98:errorcluster)  [unwired: 11 in, 1 out]
  n517 = call <userlib>:"Release Type.vi"("Handle"=w173, "TypeHandle"=w172, "error in (no error)"=w174) -> ("error out"=w185:errorcluster)  [unwired: 11 in, 1 out]
  n518 = call <userlib>:"Release Writer.vi"("Handle"=w111, "WriteHandle"=w110, "error in (no error)"=w109) -> ("error out"=w113:errorcluster)  [unwired: 11 in, 1 out]
  n519 = call <userlib>:"Release Type.vi"("Handle"=w106, "TypeHandle"=w107, "error in (no error)"=w108) -> ("error out"=w112:errorcluster)  [unwired: 11 in, 1 out]
  n520 = call <userlib>:"Release Writer.vi"("Handle"=w67, "WriteHandle"=w66, "error in (no error)"=w65) -> ("Handle"=w52:u32, "error out"=w77:errorcluster)  [unwired: 11 in]
  n521 = call <userlib>:"Release Type.vi"("Handle"=w63, "TypeHandle"=w62, "error in (no error)"=w64) -> ("error out"=w76:errorcluster)  [unwired: 11 in, 1 out]
  n522 = call <userlib>:"Release Type.vi"("Handle"=w460, "TypeHandle"=w459, "error in (no error)"=w472) -> ("error out"=w142:errorcluster)  [unwired: 11 in, 1 out]
  n523 = Merge Errors(w319, w320) -> (w130:errorcluster)
  n524 = Merge Errors(w211, w210) -> (w125:errorcluster)
  n525 = Merge Errors(w287, w286) -> (w129:errorcluster)
  n526 = Merge Errors(w249, w248) -> (w127:errorcluster)
  n527 = Merge Errors(w268, w267) -> (w128:errorcluster)
  n528 = Merge Errors(w230, w229) -> (w126:errorcluster)
  n529 = Merge Errors(w433, w434) -> (w136:errorcluster)
  n530 = Merge Errors(w325, w324) -> (w131:errorcluster)
  n531 = Merge Errors(w401, w400) -> (w135:errorcluster)
  n532 = Merge Errors(w363, w362) -> (w133:errorcluster)
  n533 = Merge Errors(w382, w381) -> (w134:errorcluster)
  n534 = Merge Errors(w344, w343) -> (w132:errorcluster)
  n535 = Merge Errors(w439, w438) -> (w137:errorcluster)
  n536 = Merge Errors(w99, w98) -> (w97:errorcluster)
  n537 = Merge Errors(w186, w185) -> (w124:errorcluster)
  n538 = Merge Errors(w113, w112) -> (w105:errorcluster)
  n539 = Merge Errors(w77, w76) -> (w61:errorcluster)
  n540 = Merge Errors(w141, w142) -> (w140:errorcluster)
  n541 = Merge Errors(w32, w31, w30, w29, w21, w2, w1) -> (w27:errorcluster)
  n542 = Merge Errors(w136, w135, w134, w133, w132, w131, w97) -> (w203:errorcluster)
  n543 = Merge Errors(w130, w129, w128, w127, w126, w125, w124, w105, w61, w15, w14, w13, w9) -> (w202:errorcluster)
  n544 = Merge Errors(w152, w153, w154, w155, w156, w58, w57, w53, w54, w55, w56) -> (w143:errorcluster)
  n545 = Merge Errors(w100, w151, w150, w149, w148, w147, w146, w145, w43, w42, w41, w28, w27) -> (w144:errorcluster)
  n546 = Merge Errors(w143, w144) -> (w8:errorcluster)
  n547 = Merge Errors(w101, w140, w137, w203, w202, w8) -> (w138:errorcluster)
  n548 = call <userlib>:"Release.vi"("Handle"=w52, "error in (no error)"=w138) -> ("error out"=→"error out":errorcluster)  [unwired: 13 in]
